vi "MainPannel.vi"() -> ()   [LabVIEW 2020]
uses:
  Digi/Digitizer_StatesMain.ctl
  <vilib>/userdefined/High Color/nirio_resource_hc.ctl
  Stage/New/StageOptions.ctl
  FileStore/Data Save State.ctl
  Gen/Generator_States.ctl
  <vilib>/Heliosphere Research LLC/Advanced Plotting Toolkit/properties/Colormap_Map.ctl
  <vilib>/Native 3D Graph/xcontrol/3DPC_SurfacePlot.xctl
  PixelImageState.ctl
  <vilib>/UPVI/lvhdf5/library.llb/HDF5 Ref.ctl
  WaveClusterPacket.ctl
  <vilib>/Platform/TimedLoop/XDataNode/timing_clust.ctl
  <vilib>/Platform/TimedLoop/XDataNode/nitl_modes.ctl
  <vilib>/Platform/TimedLoop/XDataNode/wakeup.ctl
  Stage/New/SettingCtrlOptions.ctl
  Stage/New/PosCtrlOptions.ctl
  Digi/Controls/FPGA VI Reference.ctl
  <extravilib>/ChannelInstances/Tag-bool/Read With Abort.vi
  <extravilib>/ChannelInstances/Tag-bool/Write.vi
  <extravilib>/ChannelInstances/Tag-bool/Write With Abort.vi
  <extravilib>/ChannelInstances/Tag-bool/Instantiate.vi
  <extravilib>/ChannelInstances/Tag-bool/EndpointRead.vi
  <vilib>/FPGAPlugInAG/PXIe-7962R/niLvFpga_Open_PXIe-7962R.vi
  <vilib>/rvi/interface/common/dynamic/niFpgaDynamicAddResources.vi
  <vilib>/FPGAPlugInAG/Dynamic/niLvFpga_Close_Dynamic.vi
  <extravilib>/ChannelInstances/Tag-bool/Endpoint.vi
  <instrlib>/_niInstr/Basic Elements/v1/FPGA/Private/Count Up U32.vi
  <vilib>/Platform/TimedLoop/XDataNode/XDataNode.xnode
  <vilib>/rvi/interface/nirviOpenFPGA/nirviOpenFPGA.xnode
  FPGA Bitfiles/DigitizerFPGACode(Fully_Functional)_v3.lvbitx
  <vilib>/rvi/interface/nirviCloseFPGA/nirviCloseFPGA.xnode
  <instrlib>/_niInstr/Basic Elements/v1/FPGA/niInstr Basic Elements v1 FPGA.lvlib
  <vilib>/Platform/TimedLoop/XDataNode/XDNodeRunTimeDep.lvlib
  Stage/libximc.lvlib
  <extravilib>/ChannelInstances/Tag-bool.lvlib
  <vilib>/Heliosphere Research LLC/Advanced Plotting Toolkit/Advanced Plotting Toolkit.lvlib
panel:
  in  "LogMode":bool
  in  "Start Digitizer UI Bttn":bool
  out "Max Index (s)":dbl format="%#_3p"
  out "Max Val (V)":dbl format="%#_3p"
  in  "Delay_Scroll_Range":dbl=2.0 caption="Range"
  in  "FineDelayControl":dbl(slide)=1.0 step=0.1 scale=-2.0..2.0
  in  "Amplitude Range":cluster{"Slider 1":dbl, "Slider 1":dbl}(slide)={"Slider 1"=1.0, "Slider 1"=1.6299559471365639} scale=-2.5..2.5
  in  "Pause Triggger":bool caption="Pause"
  in  "Delay(us)":sgl min=0 step=0.1 format="%#_4g"
  in  "Time Division":u8(slide)=1 max=2 step=1 scale=0.0..2.0
  in  "Amplitude \nAveraging":u16(slide)=1 caption="Amplitude Averaging" scale=0.0..7.0 scale format="%#.2g"
  in  "Record Size":u16=1024
  in  "RIO Resource":T1="PXI1Slot2"
  out "Configured?":bool
  out "TIS Configured?":bool
  out "Range (Vpp)":dbl=1.3
  out "Digitizer On":bool
  out "Waveform [LIVE]":cluster{"Start Time":dbl, dbl, ext[]}(graph)
  in  "TriggerDigi":bool
  in  "Scanning":bool
  in  "Single Shot":bool
  in  "LIVE":bool
  out "Topography Plot":refnum<class "Base Datatype.lvclass">[](xcontrol)
  in  "Axis":bool
  in  "ColorBar":bool
  in  "Map":T2
  out "Scanned Image":picture
  in  "Transducer Freq (Hz)":u64
  in  "Temperature (C)":dbl
  in  "Remarks":string
  in  "Immersion Medium":string
  in  "EXIT APP":bool
  in  "Save to File":bool=TRUE caption="Checkbox"
  out "No Trig Miss":bool
  in  "FileName":string
  in  "File Store Directory":path
  out "File Open?":bool
  out "X Step Size (R)":sgl format="%#_2g"
  out "Y Step Size (R)":sgl format="%#_2g"
  out "Scan Time (Approx.)":string
  out "Total Pixels":i32
  out "Moving?":bool
  out "Stage Position":cluster{sgl[], sgl[]}(graph) caption="XY Graph - Dark"
  in  "X Position Abs":dbl caption="X Position"
  in  "Y Position Abs":dbl caption="Y Position"
  out "Line Count":i32=6 caption="Y Pixels"
  out "Pixel Count":i32=6 caption="X Pixels"
  in  "X Start":sgl
  in  "X End":sgl=10.0
  in  "Y Start":sgl
  in  "Y End":sgl=8.0
  in  "Y Step Size":sgl=0.5
  in  "X Step Size":sgl=0.5
  in  "Scan Mode":enum16{"Raster", "Serpentine"}(ring)
  in  "Speed Control (mm/s)":sgl(slide)=4.0 min=0.1 scale=0.1..5.0
  in  "AbsMove":bool
  in  "Outline":bool
  in  "Start Stage":bool
  in  "Stop Motion":bool
  in  "Zero":bool
  in  "Right":bool
  in  "Left":bool
  in  "Move to Start":bool
  in  "Down":bool
  in  "Up":bool
  out "X Position":dbl format="%#.3g"
  out "Y Position":dbl format="%#.3g"
  in  "Move Step":dbl=1.0
  in  "Stop Stage":bool
  out "Controller Open?":bool
  in  "Tab Control":enum32{"Developer Options"}(tab)
  out "Scan Running":bool=TRUE
  in  "Next Coordinate Index":i32
  in  "EdgePt/nPixelMap":bool=TRUE
  out "Coordinate Array":sgl[][](array[numeric])
  out "Step Sizes":sgl[](array[numeric])
  out "Peripheral Coordis":sgl[][](array[numeric])=[[0.0, 0.0], [1.8, 0.0], [3.6, 0.0], [5.3999996, 0.0], [7.2, 0.0], [9.0, 0.0], [9.0, 2.0], [7.2, 2.0], [5.3999996, 2.0], [3.6, 2.0], [1.8, 2.0], [0.0, 2.0], [0.0, 4.0], [1.8, 4.0], [3.6, 4.0], [5.3999996, 4.0], [7.2, 4.0], [9.0, 4.0], [9.0, 6.0], [7.2, 6.0], [5.3999996, 6.0], [3.6, 6.0], [1.8, 6.0], [0.0, 6.0], [0.0, 8.0], [1.8, 8.0], [3.6, 8.0], [5.3999996, 8.0], [7.2, 8.0], [9.0, 8.0], [9.0, 10.0], [7.2, 10.0], [5.3999996, 10.0], [3.6, 10.0], [1.8, 10.0], [0.0, 10.0]]
  in  "Correction Table Path (Hidden)":path
  out "Serial nos":u32[](array[numeric])
  out "Calibration":cluster{dbl, "MicrostepMode":u32}[](array[cluster])
  out "IDs":i32[](array[numeric])
  in  "X Max Stage":dbl=220.0 format="%#_13g"
  in  "Y Maximum":dbl=220.0
  out "Stage Status":T3
  out "Waves Received":u32
  in  "reset Rx wave count":bool
  out "Digi State":T4
  out "nDigiLoopRunning":bool
  in  "Send vi Trig":bool
  out "Gain":dbl
  out "Offset Factor":dbl
  out "Amplitudes":dbl[](array[numeric]) format="%.2f"
  out "Sampling Frequency (Hz)":u64
  out "Waves per Pixel":u32
  in  "Ext/nViTrig":bool=TRUE
  out "FileStore State":T5
  out "Gen State":T6
  out "PixelMap_Scan":i32[][](array[numeric])
  out "error out Digi":errorcluster
  in  "Scan Started":bool
  out "Scan Complete":bool=TRUE
  out "Image State":T7
  out "Wave Count Zero":bool
  out "Error Out Gen":errorcluster
  in  "CountReset":bool
  in  "Stop Gen App":bool
  in  "Machine Mode":T8(ring)=enum."Normal"
  in  "Stop Stage App":bool
  in  "Trigger Digi Single":bool
  in  "Start Digi":bool
  in  "Stop Digi App":bool caption="Stop Digi \nApplication"
  in  "Digi Machine Mode":T9(ring)=enum."Single Shot Mode"
  in  "Done Recording":bool
  in  "Record Data":bool
  in  "Open File":bool
  in  "Stop File App":bool
  in  "Reset Img Ma":bool
  in  "Generator  Port":refnum<k15>
  out "Actual Sample Rate":dbl format="%#_6p"
  in  "Use Default Wave Settings":bool caption="Checkbox"
  in  "Start Gen":bool
  in  "stop Gen":bool
  out "Generator On":bool
  out "Input Waveform":dbl[](graph)
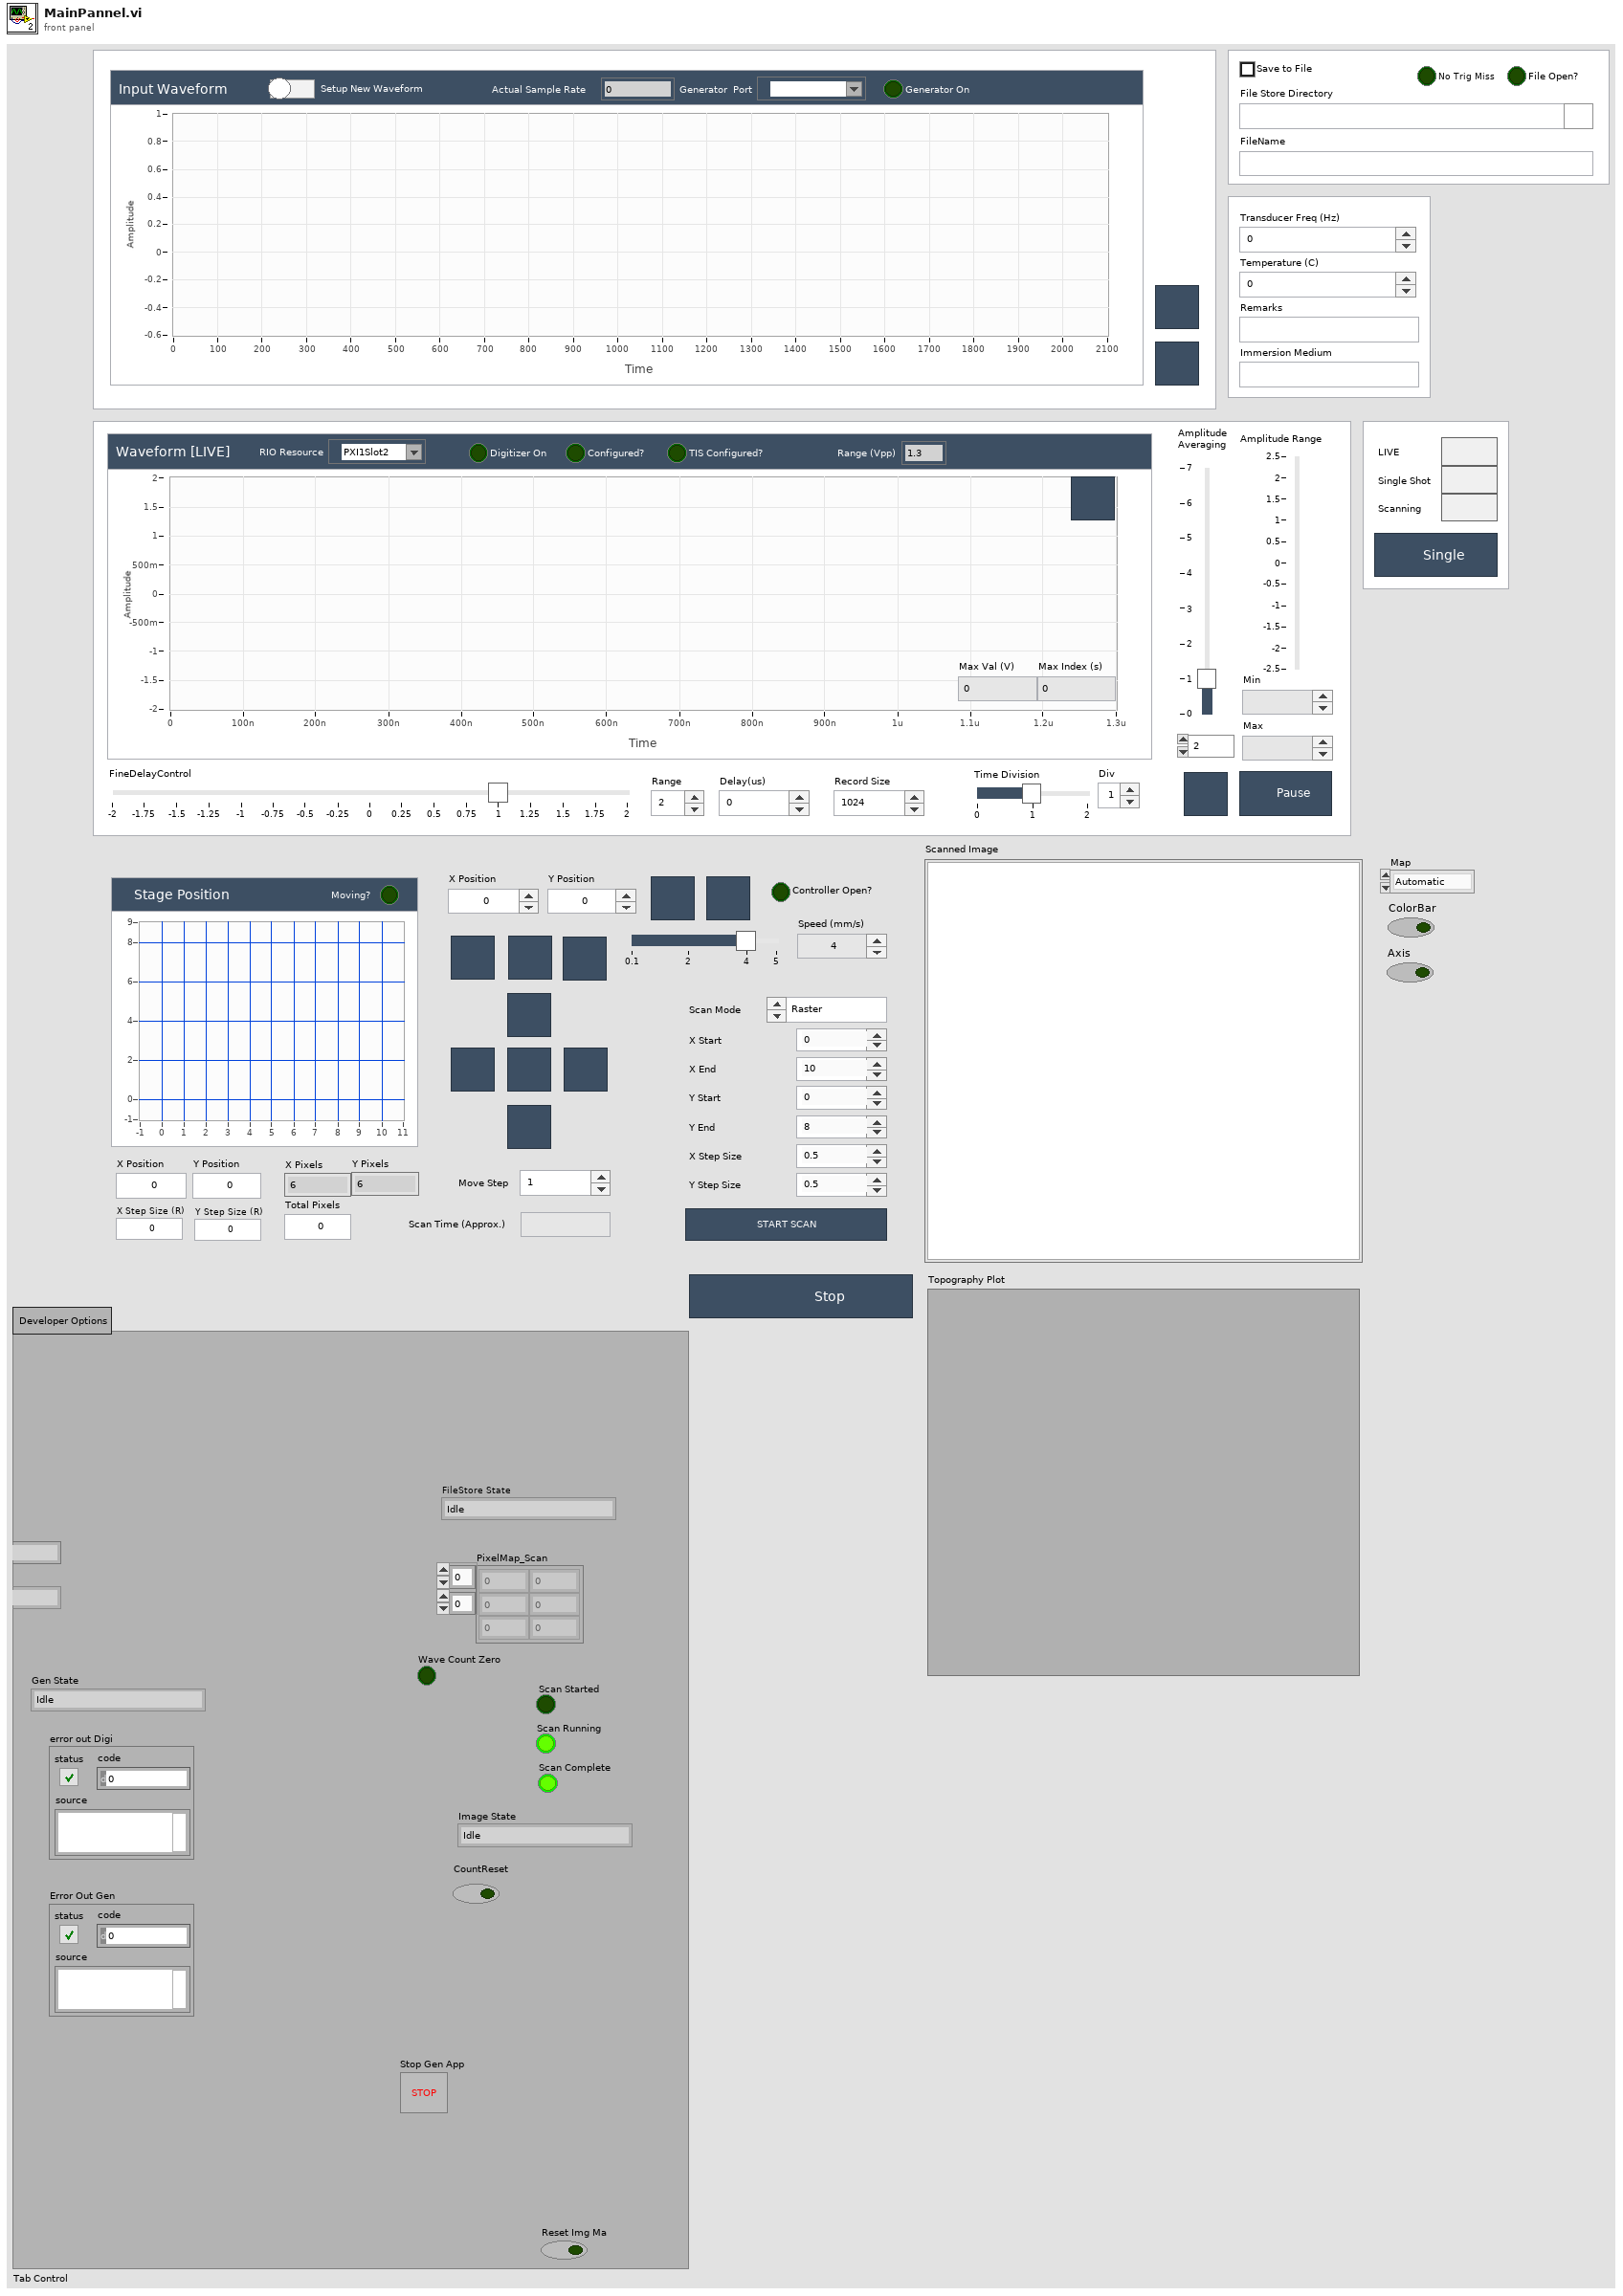
[diagram p1: front panel]
types:
  T1 = typedef "nirio_resource_hc.ctl" = tag
  T2 = typedef "Advanced Plotting Toolkit.lvlib/Colormap_Map.ctl" = enum16{"Automatic", "Rainbow", "Hot and Cold", "White-Black", "White-Blue", "White-Green", "White-Red", "Fire", "Water", "Earth", "Air", "Pastel", "Banded", "Stepped"}
  T3 = typedef "StageOptions.ctl" = enum16{"Idle", "Init", "Set Speed", "GenerateMotionPoints", "Scan_Start", "Scan_MoveNext", "Scan_SyncSet", "Scan_Get Pos", "Scan_Complete", "Cmd_MoveAbs", "Cmd_CloseControllers", "Cmd_MoveUp", "Cmd_MoveDown", "Cmd_MoveLeft", "Cmd_MoveRight", "Cmd_MoveStart", "Cmd_MoveZero", "Cmd_GetPos", "Cmd_Stop", "Sync_On", "Sync_Off", "Stop Motion", "CloseApplication"}
  T4 = typedef "Digitizer_StatesMain.ctl" = enum16{"Idle", "Init", "SetParam", "VITrig", "Read", "CloseDigi", "CloseApp"}
  T5 = typedef "Data Save State.ctl" = enum16{"Idle", "Open File", "Write Attributes", "Append Data", "Close File", "Close App"}
  T6 = typedef "Generator_States.ctl" = enum16{"Idle", "GenerateWaveArray", "InitGen", "SendVITrig", "CloseGen", "CloseApp"}
  T7 = typedef "PixelImageState.ctl" = enum16{"Idle", "Init", "Update Pixel", "Complete Imaging"}
  T8 = enum16{"Scanning Mode", "Perimeter Mode", "Normal"}
  T9 = enum16{"Scanning Mode", "Live Mode", "Single Shot Mode"}
  T10 = typedef "WaveClusterPacket.ctl" = cluster{"Wave Count":u32, "Wave":i16[]}
  T11 = typedef "HDF5 Ref.ctl" = refnum<k1>
  T12 = typedef "XDNodeRunTimeDep.lvlib/timing_clust.ctl" = cluster{"Expected End [f-1]":u64, "Actual End [f-1]":u64, "Finished Late? [f-1]":bool, "Expected End [i-1]":u64, "Actual End [i-1]":u64, "Finished Late? [i-1]":bool, "Expected Start [i]":u64, "Actual Start [i]":u64, "Expected Start [f]":u64, "Actual Start [f]":u64, "Source Name":string, "Structure Name":string, "Period":i64, "Deadline":i64, "Offset":i64, "Start":i64, "Priority":i32, "Timeout":i32, "Mode":T13, "Wakeup Reason":T14, "Error":errorcluster, "Source Type":string, "Secondary Source Type":string, "Global End Time":u64, "Global Start Time":u64, "Frame Duration":u64, "Iteration Duration":u64, "Assigned CPU":i32, "I/O Scan Engine Mode":u32}
  T13 = typedef "XDNodeRunTimeDep.lvlib/nitl_modes.ctl" = enum32{"No Change", "Process missed periods, maintain original phase", "Discard missed periods, maintain original phase", "Process missed periods, ignore original phase", "Discard missed periods, ignore original phase"}
  T14 = typedef "XDNodeRunTimeDep.lvlib/wakeup.ctl" = enum32{"Normal", "Aborted", "Asynchronous wakeup", "Timing source error", "Timed loop error", "Timeout"}
  T15 = typedef "SettingCtrlOptions.ctl" = enum16{"Set X", "Set Y", "Set X and Y", "Get Settings", "None"}
  T16 = typedef "PosCtrlOptions.ctl" = enum16{"Move X", "Move Y", "Both X and Y", "Read Pos", "None"}
  T17 = typedef "FPGA VI Reference.ctl" = refnum<k20>
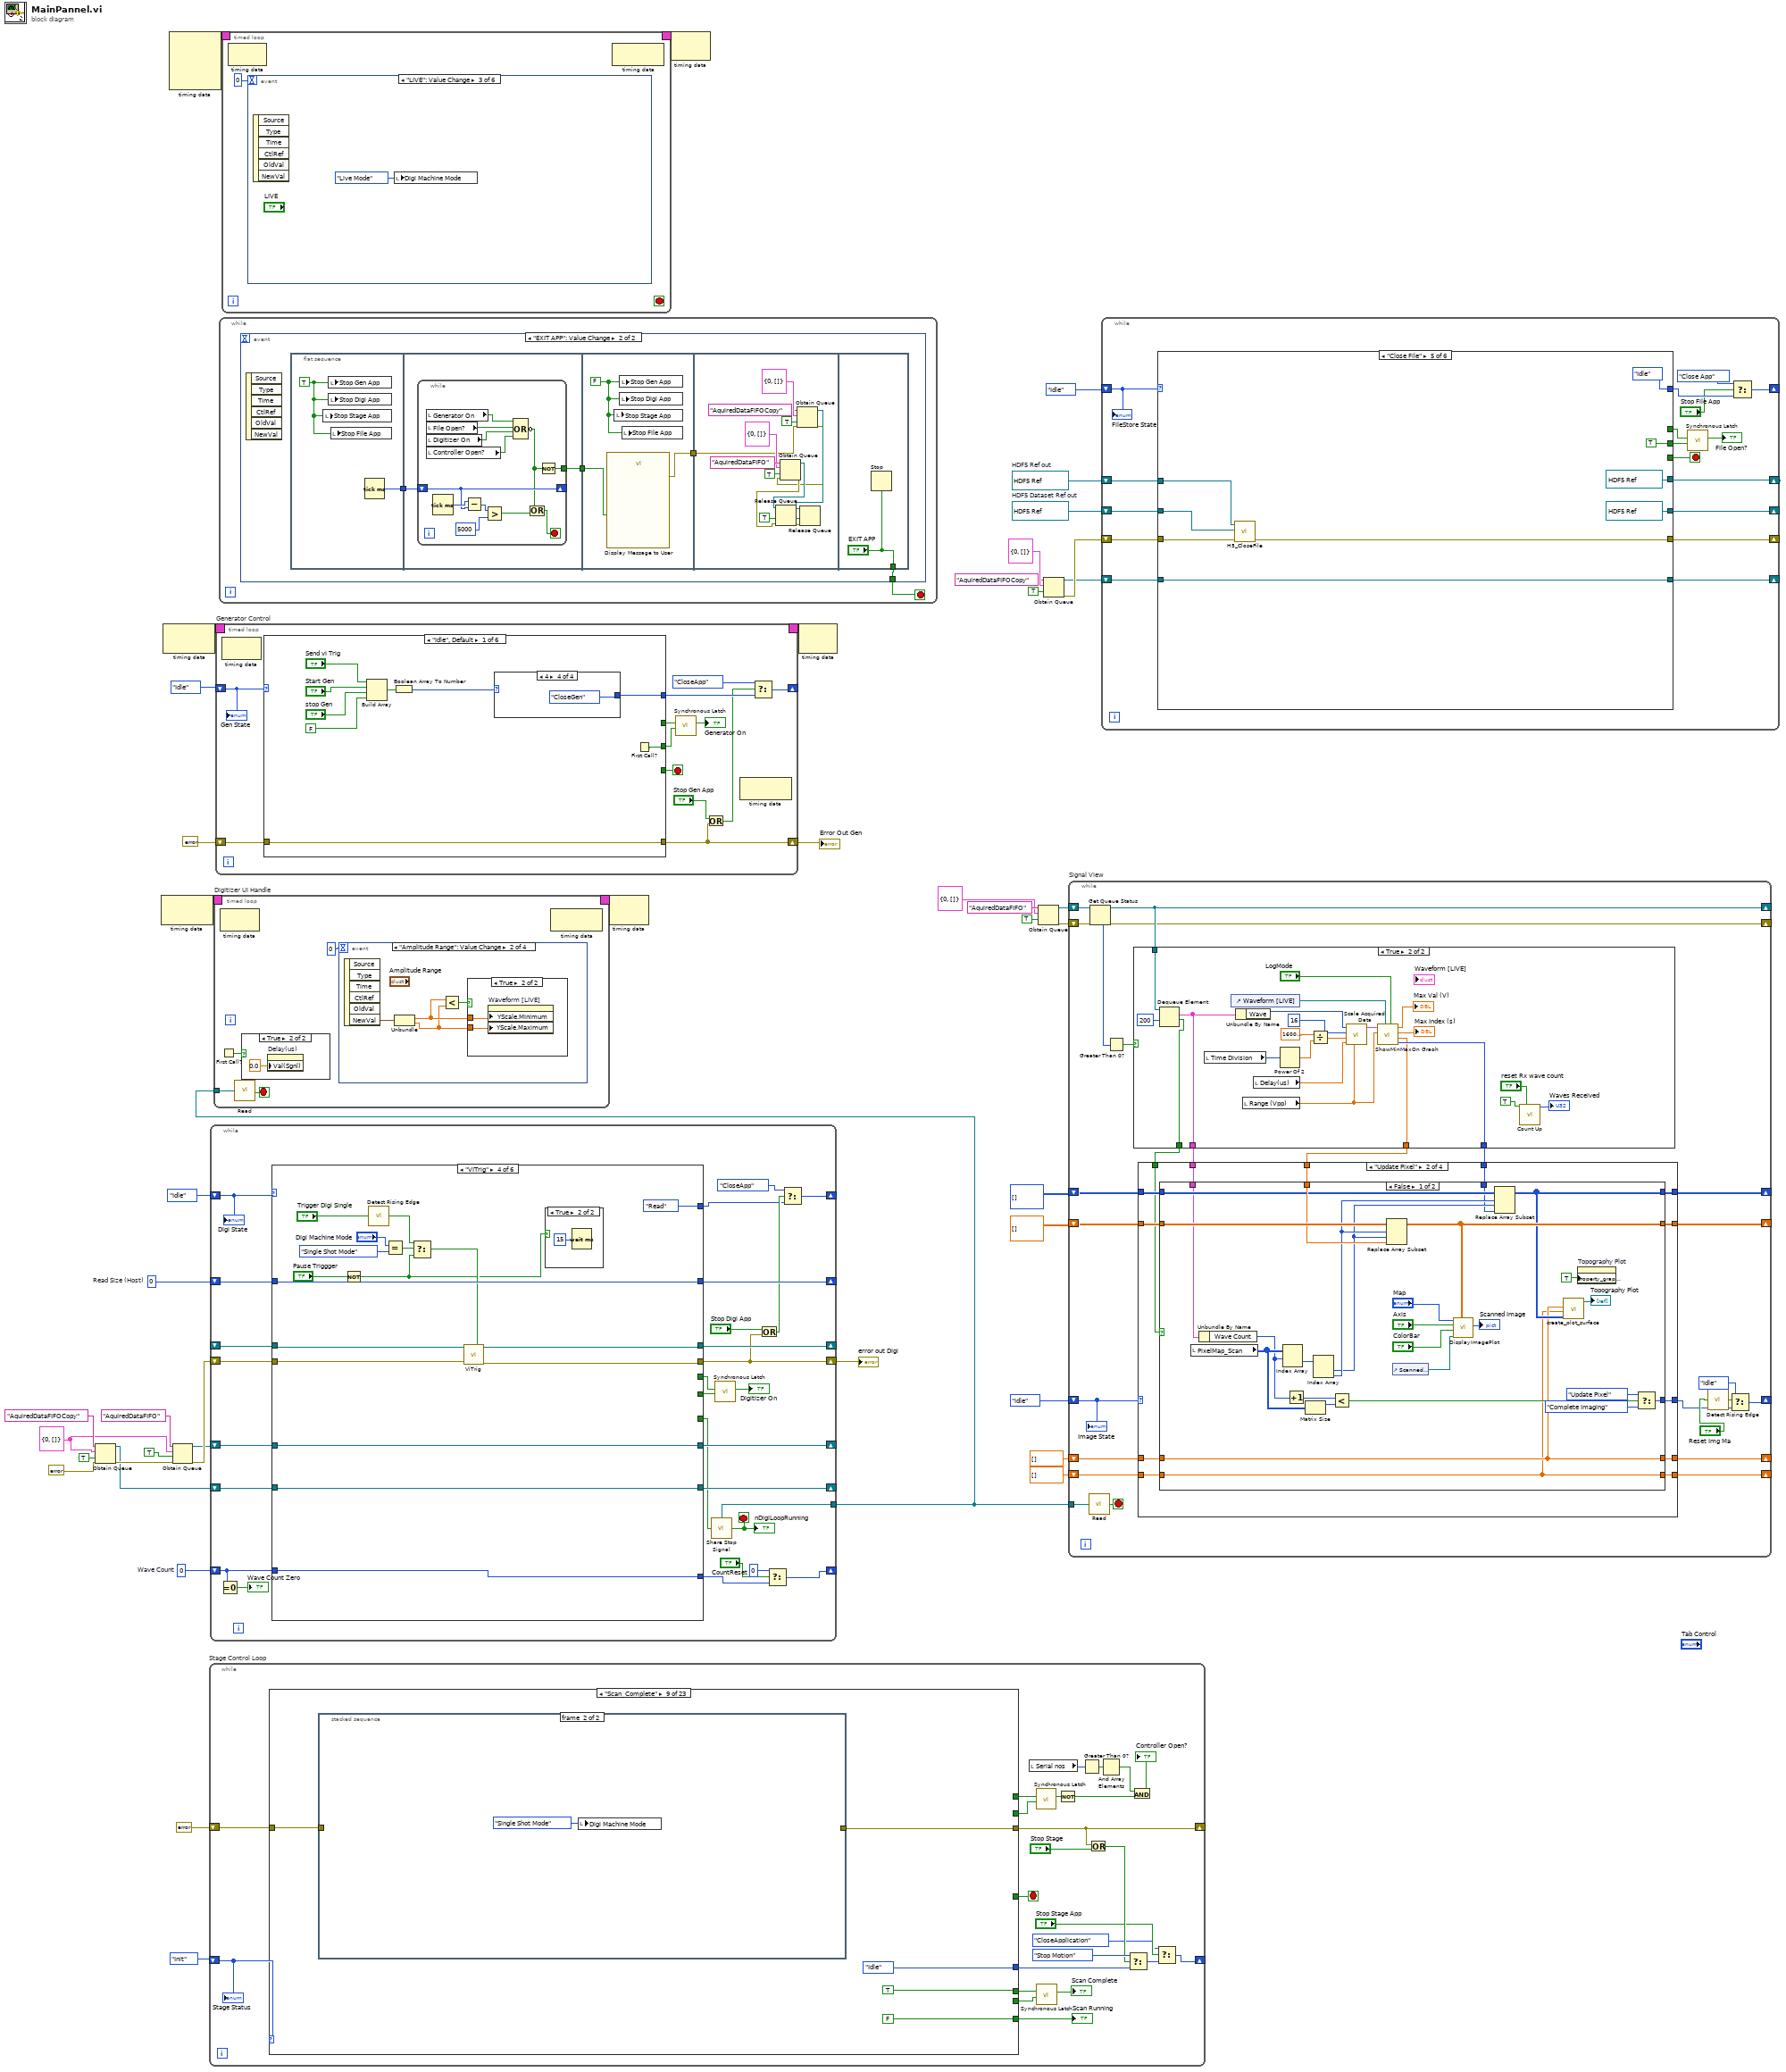
[diagram p0: block diagram]
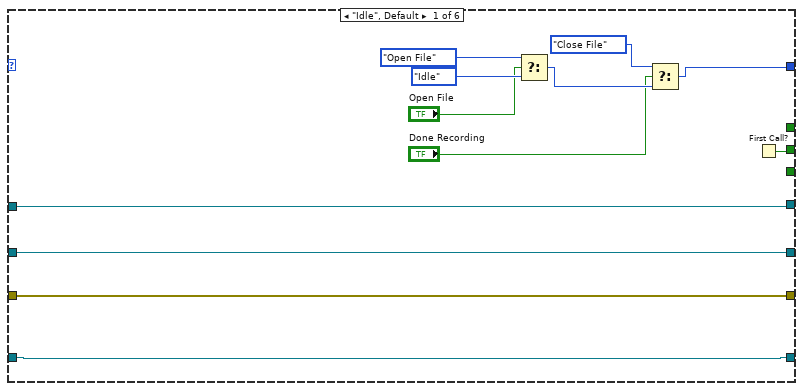
[diagram p2: hidden frame]
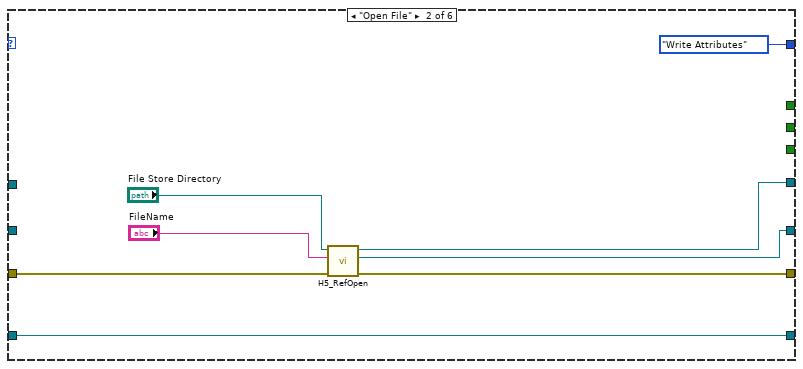
[diagram p3: hidden frame]
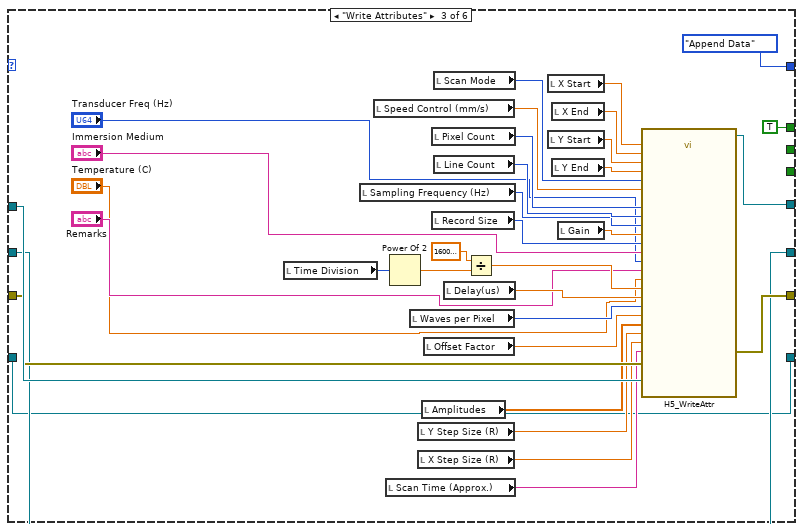
[diagram p4: hidden frame]
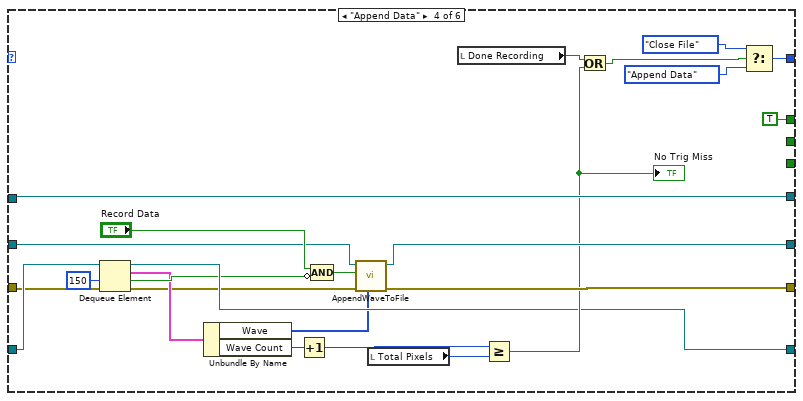
[diagram p5: hidden frame]
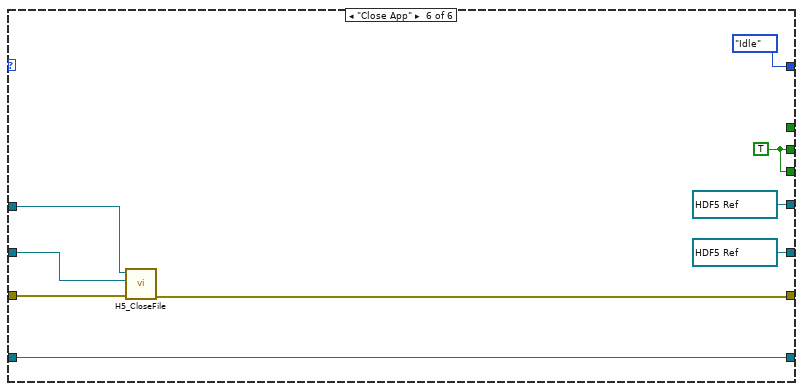
[diagram p6: hidden frame]
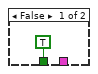
[diagram p7: hidden frame]
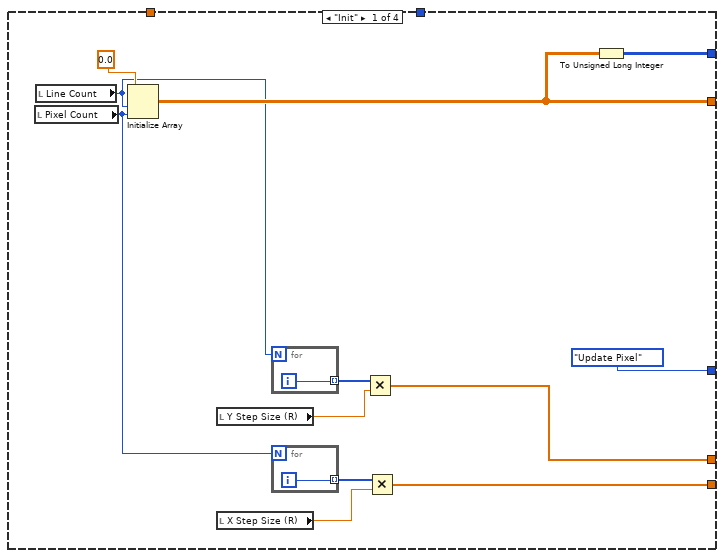
[diagram p8: hidden frame]
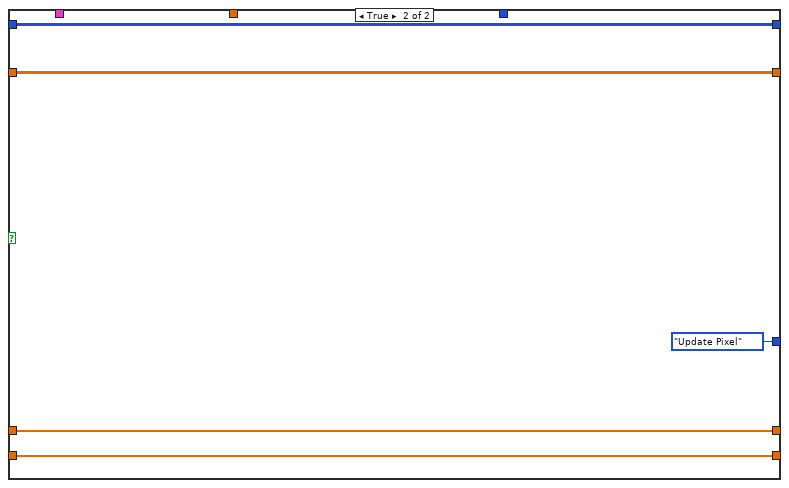
[diagram p9: hidden frame]
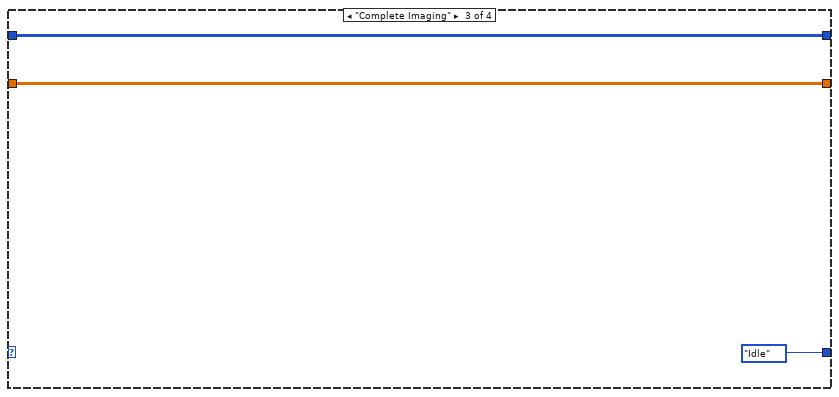
[diagram p10: hidden frame]
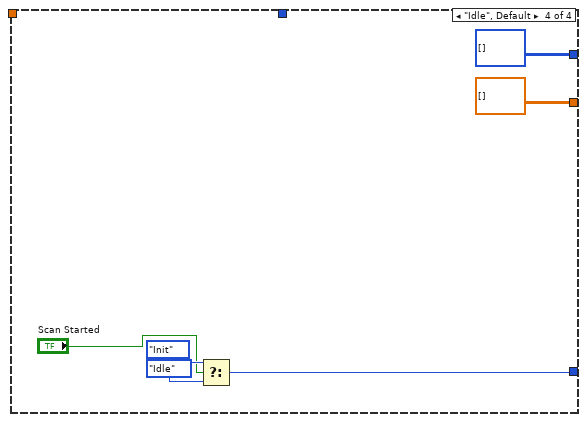
[diagram p11: hidden frame]
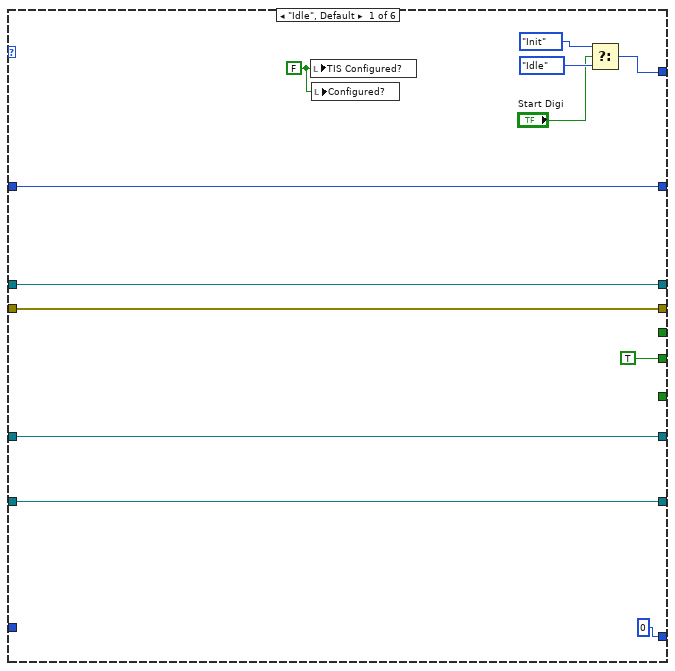
[diagram p12: hidden frame]
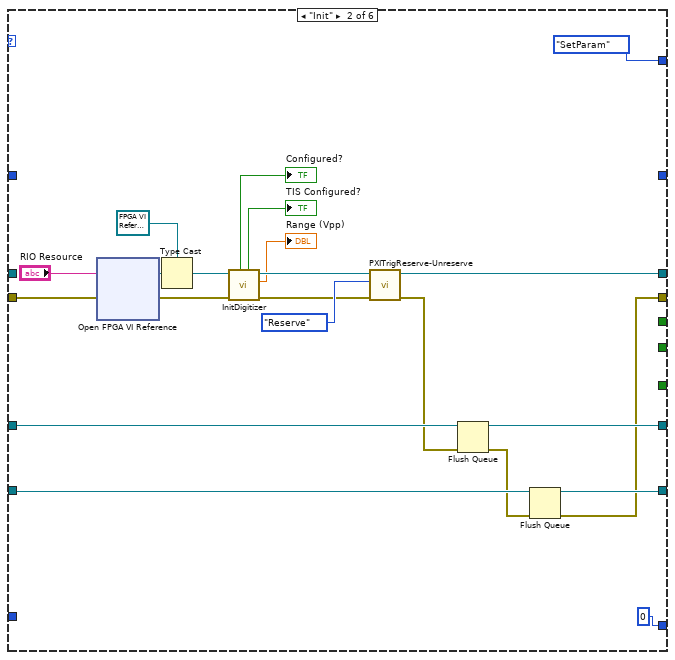
[diagram p13: hidden frame]
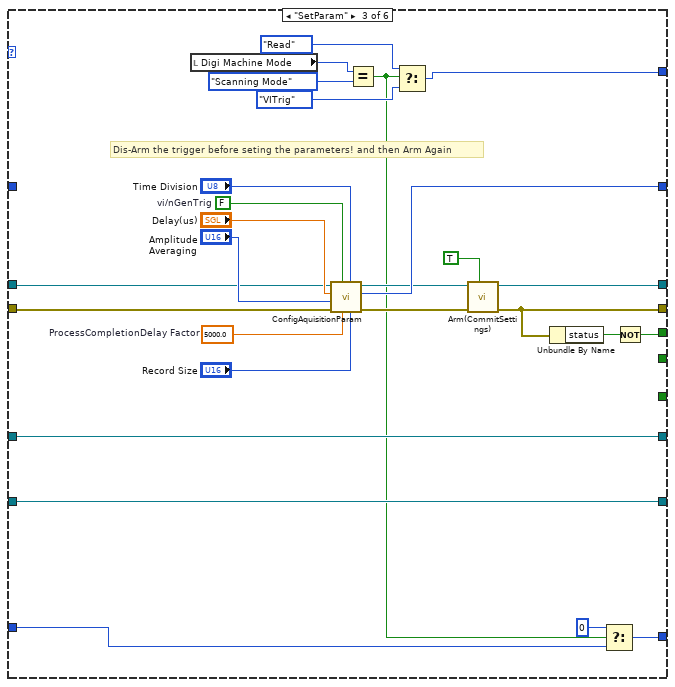
[diagram p14: hidden frame]
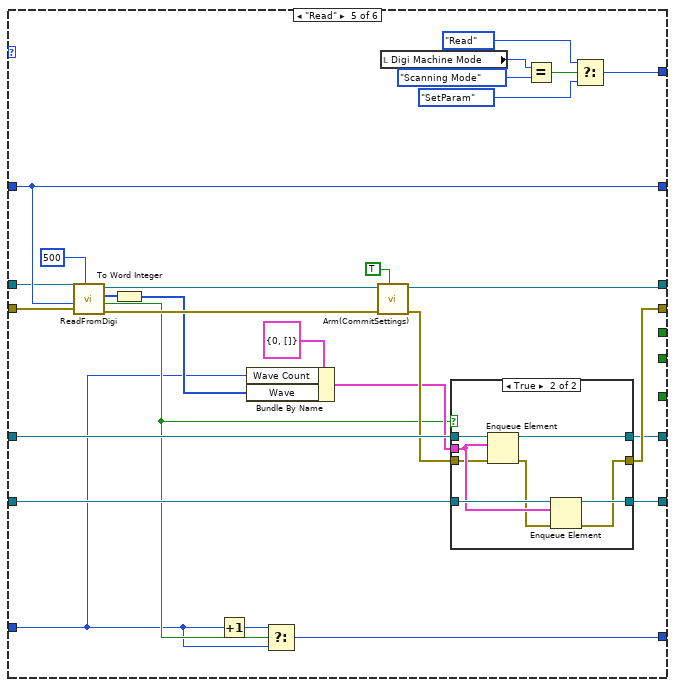
[diagram p16: hidden frame]
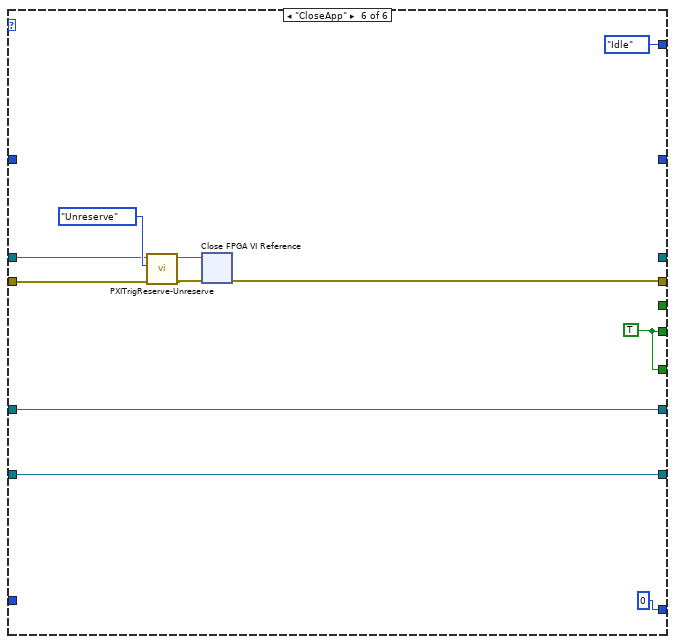
[diagram p18: hidden frame]
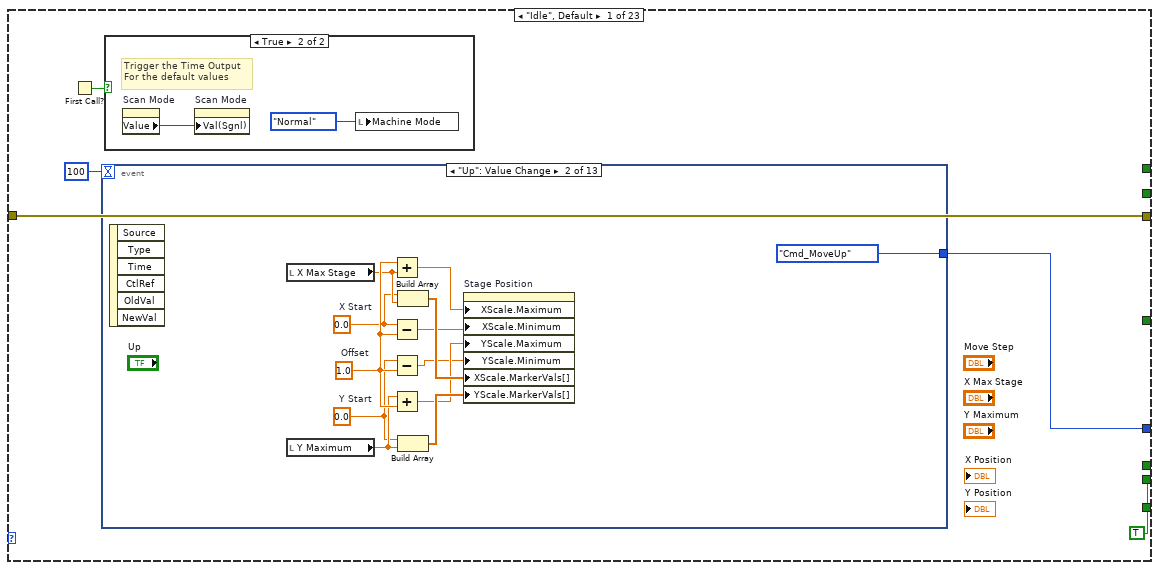
[diagram p19: hidden frame]
diagram:
  w12 = u16 0  # Wave Count
  w14 = T10 {"Wave Count"=0, "Wave"=[]} ("input cluster")
  w21 = T11 refnum items=["HDF5 Ref"]  # HDF5 Dataset Ref out
  w22 = T11 refnum items=["HDF5 Ref"]  # HDF5 Ref out
  w39 = u16 0  # Read Size (Host)
  n1 = Obtain Queue(name (unnamed)="AquiredDataFIFOCopy", element data type=w14, create if not found? (T)=TRUE, error in (no error)=errorcluster {"status"=FALSE, "code"=0, "source"=""}) -> (queue out=w16:refnum<queue>, error out=w17:errorcluster)  [unwired: 1 in, 1 out]
  n2 = node-c288() -> (w42:T12)  [unwired: 1 in]
  n3 = node-c288() -> (w36:T12)  [unwired: 1 in]
  n4 = node-c288() -> (w5:T12)  [unwired: 4 in]
  n5 = Obtain Queue(name (unnamed)="AquiredDataFIFO", element data type=w14, create if not found? (T)=TRUE, error in (no error)=w17) -> (queue out=w28:refnum<queue>, error out=w29:errorcluster)  [unwired: 1 in, 1 out]
  n6 = while "Stage Control Loop" {
    shift-right: [w57] -> _
    shift-left: StageOptions."Init" -> [w68]
    shift-right: [w65] -> _
    shift-left: errorcluster {"status"=FALSE, "code"=0, "source"=""} ("error out") -> [w66]
    stop <- w58 stop-if-true
    n7 = case shown="\"Scan_Complete\"" w68 {
      tunnel: [w73 w169 w192 w228 w233 w362 w377 w391 w431 w454 w463 w470 w481 w491 w501 w510 w518 w533 w539 w550 w559 w567 w578] -> w65
      tunnel: w66 -> [w73 w167 w193 w227 w235 w363 w378 w392 w429 w455 w464 w469 w482 w492 w502 w511 w519 w534 w538 w551 w560 w566 w577]
      tunnel: [w72 StageOptions."Set Speed" StageOptions."GenerateMotionPoints" w212 w236 w353 StageOptions."Scan_MoveNext" w388 StageOptions."Idle" StageOptions."Idle" StageOptions."Idle" StageOptions."Idle" StageOptions."Idle" StageOptions."Idle" StageOptions."Idle" StageOptions."Idle" StageOptions."Idle" StageOptions."Idle" StageOptions."Idle" StageOptions."Idle" StageOptions."Idle" StageOptions."Idle" StageOptions."Idle"] -> w63
      tunnel: [_ _ _ _ _ _ _ _ _ _ _ _ _ _ _ _ _ _ _ _ _ w563 w573] -> w61
      tunnel: [_ w170 _ _ _ _ _ _ _ _ _ _ _ _ _ _ _ _ _ _ _ _ _] -> w59
      tunnel: [_ _ _ _ _ _ _ _ _ _ _ _ _ _ _ _ _ _ _ _ _ _ w573] -> w58
      tunnel: [_ _ _ _ _ _ _ _ TRUE ("X SyncOut Enabled") _ _ _ _ _ _ _ _ _ _ _ _ _ _] -> w48
      tunnel: [TRUE ("EdgePt/nPixelMap") TRUE ("EdgePt/nPixelMap") TRUE ("EdgePt/nPixelMap") TRUE ("EdgePt/nPixelMap") TRUE ("EdgePt/nPixelMap") _ _ _ _ _ _ _ _ _ _ _ _ _ _ _ _ _ _] -> w46
      tunnel: [_ _ _ _ _ TRUE ("Moving?") TRUE ("Moving?") w379 FALSE ("Moving?") _ _ _ _ _ _ _ _ _ _ _ _ _ _] -> w45
      frame "Idle", Default {
        n8 = First Call?() -> (First Call?: T/F=w70:bool)
        n9 = event shown="[1] \"Up\": Value Change" {
          selector: _ -> [_ _ _ _ _ _ _ _ _ _ _ _ _]
          dyn-events: _ -> [_ _ _ _ _ _ _ _ _ _ _ _ _]
          timeout: 100 -> [_ _ _ _ _ _ _ _ _ _ _ _ _]
          tunnel: [w76 StageOptions."Cmd_MoveUp" StageOptions."Cmd_MoveDown" StageOptions."Cmd_MoveStart" StageOptions."Cmd_MoveLeft" StageOptions."Cmd_MoveRight" StageOptions."Cmd_MoveZero" StageOptions."Cmd_Stop" StageOptions."GenerateMotionPoints" StageOptions."GenerateMotionPoints" StageOptions."Set Speed" w148 StageOptions."Cmd_MoveAbs"] -> w72
          event Timeout {
            n10 = event-data() -> ()  [unwired: 1 in, 3 out]
            n11 = local read "Controller Open?"() -> (w77:bool)
            n12 = case shown="False" w77 {
              tunnel: [StageOptions."Init" StageOptions."Cmd_GetPos"] -> w76
              frame False {
              }
              frame True {
              }
            }
          }
          event "Up": Value Change {
            w80 = 0.0  # Y Start
            w82 = sgl 0.0  # X Start
            w85 = 1.0  # Offset
            n13 = event-data() -> ()  [unwired: 1 in, 6 out]
            n14 = local read "X Max Stage"() -> (w83:dbl)
            n15 = local read "Y Maximum"() -> (w81:dbl)
            n16 = Add(x=w85, y=w83) -> (x+y=w87:dbl)
            n17 = Subtract(x=w82, y=w85) -> (x-y=w88:dbl)
            n18 = Subtract(x=w80, y=w85) -> (x-y=w84:dbl)
            n19 = Add(x=w81, y=w85) -> (x+y=w86:dbl)
            n20 = Build Array(w82, w83) -> (w90:dbl[])
            n21 = Build Array(w80, w81) -> (w89:dbl[])
            n22 = property on="Stage Position" class="XYGraph (strict)"("XScale.Maximum"=w87, "XScale.Minimum"=w88, "YScale.Maximum"=w86, "YScale.Minimum"=w84, "XScale.MarkerVals[]"=w90, "YScale.MarkerVals[]"=w89) -> ()  [unwired: 2 in, 2 out]
          }
          event "Down": Value Change {
            w92 = 0.0  # Y Start
            w94 = sgl 0.0  # X Start
            w97 = 1.0  # Offset
            n23 = event-data() -> ()  [unwired: 1 in, 6 out]
            n24 = local read "X Max Stage"() -> (w95:dbl)
            n25 = local read "Y Maximum"() -> (w93:dbl)
            n26 = Add(x=w97, y=w95) -> (x+y=w99:dbl)
            n27 = Subtract(x=w94, y=w97) -> (x-y=w100:dbl)
            n28 = Subtract(x=w92, y=w97) -> (x-y=w96:dbl)
            n29 = Add(x=w93, y=w97) -> (x+y=w98:dbl)
            n30 = Build Array(w94, w95) -> (w102:dbl[])
            n31 = Build Array(w92, w93) -> (w101:dbl[])
            n32 = property on="Stage Position" class="XYGraph (strict)"("XScale.Maximum"=w99, "XScale.Minimum"=w100, "YScale.Maximum"=w98, "YScale.Minimum"=w96, "XScale.MarkerVals[]"=w102, "YScale.MarkerVals[]"=w101) -> ()  [unwired: 2 in, 2 out]
          }
          event "Move to Start": Value Change {
            n33 = event-data() -> ()  [unwired: 1 in, 6 out]
          }
          event "Left": Value Change {
            w105 = 0.0  # Y Start
            w107 = sgl 0.0  # X Start
            w110 = 1.0  # Offset
            n34 = event-data() -> ()  [unwired: 1 in, 6 out]
            n35 = local read "X Max Stage"() -> (w108:dbl)
            n36 = local read "Y Maximum"() -> (w106:dbl)
            n37 = Add(x=w110, y=w108) -> (x+y=w112:dbl)
            n38 = Subtract(x=w107, y=w110) -> (x-y=w113:dbl)
            n39 = Subtract(x=w105, y=w110) -> (x-y=w109:dbl)
            n40 = Add(x=w106, y=w110) -> (x+y=w111:dbl)
            n41 = Build Array(w107, w108) -> (w115:dbl[])
            n42 = Build Array(w105, w106) -> (w114:dbl[])
            n43 = property on="Stage Position" class="XYGraph (strict)"("XScale.Maximum"=w112, "XScale.Minimum"=w113, "YScale.Maximum"=w111, "YScale.Minimum"=w109, "XScale.MarkerVals[]"=w115, "YScale.MarkerVals[]"=w114) -> ()  [unwired: 2 in, 2 out]
          }
          event "Right": Value Change {
            w117 = 0.0  # Y Start
            w119 = sgl 0.0  # X Start
            w122 = 1.0  # Offset
            n44 = event-data() -> ()  [unwired: 1 in, 6 out]
            n45 = local read "X Max Stage"() -> (w120:dbl)
            n46 = local read "Y Maximum"() -> (w118:dbl)
            n47 = Add(x=w122, y=w120) -> (x+y=w124:dbl)
            n48 = Subtract(x=w119, y=w122) -> (x-y=w125:dbl)
            n49 = Subtract(x=w117, y=w122) -> (x-y=w121:dbl)
            n50 = Add(x=w118, y=w122) -> (x+y=w123:dbl)
            n51 = Build Array(w119, w120) -> (w127:dbl[])
            n52 = Build Array(w117, w118) -> (w126:dbl[])
            n53 = property on="Stage Position" class="XYGraph (strict)"("XScale.Maximum"=w124, "XScale.Minimum"=w125, "YScale.Maximum"=w123, "YScale.Minimum"=w121, "XScale.MarkerVals[]"=w127, "YScale.MarkerVals[]"=w126) -> ()  [unwired: 2 in, 2 out]
          }
          event "Zero": Value Change {
            w129 = 0.0  # Y Start
            w131 = sgl 0.0  # X Start
            w134 = 1.0  # Offset
            n54 = event-data() -> ()  [unwired: 1 in, 6 out]
            n55 = local read "X Max Stage"() -> (w132:dbl)
            n56 = local read "Y Maximum"() -> (w130:dbl)
            n57 = Add(x=w134, y=w132) -> (x+y=w136:dbl)
            n58 = Subtract(x=w131, y=w134) -> (x-y=w137:dbl)
            n59 = Subtract(x=w129, y=w134) -> (x-y=w133:dbl)
            n60 = Add(x=w130, y=w134) -> (x+y=w135:dbl)
            n61 = Build Array(w131, w132) -> (w139:dbl[])
            n62 = Build Array(w129, w130) -> (w138:dbl[])
            n63 = property on="Stage Position" class="XYGraph (strict)"("XScale.Maximum"=w136, "XScale.Minimum"=w137, "YScale.Maximum"=w135, "YScale.Minimum"=w133, "XScale.MarkerVals[]"=w139, "YScale.MarkerVals[]"=w138) -> ()  [unwired: 2 in, 2 out]
          }
          event "Stop Motion": Value Change {
            n64 = event-data() -> ()  [unwired: 1 in, 6 out]
          }
          event "Start Stage": Value Change {
            n65 = event-data() -> ()  [unwired: 1 in, 6 out]
            n66 = local write "Machine Mode"(T8."Scanning Mode" ("Machine Mode")) -> ()
          }
          event "X Start", "X End", "Y Start", "Y End", "Y Step Size", "X Step Size", "Scan Mode": Value Change {
            n67 = event-data() -> ()  [unwired: 1 in, 6 out]
            n68 = local write "Machine Mode"(T8."Normal" ("Machine Mode")) -> ()
          }
          event "Speed Control (mm/s)": Value Change {
            n69 = event-data() -> ()  [unwired: 1 in, 6 out]
          }
          event "Outline": Value Change {
            n70 = event-data() -> ()  [unwired: 1 in, 6 out]
            n71 = case shown="True" "Outline" {
              tunnel: [StageOptions."Idle" StageOptions."GenerateMotionPoints"] -> w148
              frame False {
              }
              frame True {
                n72 = local write "Machine Mode"(T8."Perimeter Mode" ("Machine Mode")) -> ()
              }
            }
          }
          event "AbsMove": Value Change {
            w152 = 0.0  # Y Start
            w154 = sgl 0.0  # X Start
            w157 = 1.0  # Offset
            n73 = event-data() -> ()  [unwired: 1 in, 6 out]
            n74 = local read "X Max Stage"() -> (w155:dbl)
            n75 = local read "Y Maximum"() -> (w153:dbl)
            n76 = Add(x=w157, y=w155) -> (x+y=w159:dbl)
            n77 = Subtract(x=w154, y=w157) -> (x-y=w160:dbl)
            n78 = Subtract(x=w152, y=w157) -> (x-y=w156:dbl)
            n79 = Add(x=w153, y=w157) -> (x+y=w158:dbl)
            n80 = Build Array(w154, w155) -> (w162:dbl[])
            n81 = Build Array(w152, w153) -> (w161:dbl[])
            n82 = property on="Stage Position" class="XYGraph (strict)"("XScale.Maximum"=w159, "XScale.Minimum"=w160, "YScale.Maximum"=w158, "YScale.Minimum"=w156, "XScale.MarkerVals[]"=w162, "YScale.MarkerVals[]"=w161) -> ()  [unwired: 2 in, 2 out]
          }
        }
        n83 = case shown="True" w70 {
          frame False {
          }
          frame True {
            # "Trigger the Time Output\nFor the default values"
            n84 = property on="Scan Mode" class="Enum (strict)"() -> ("Value"=w75:enum16{"Raster", "Serpentine"})  [unwired: 2 in, 2 out]
            n85 = property on="Scan Mode" class="Enum (strict)"("Val(Sgnl)"=w75) -> ()  [unwired: 2 in, 2 out]
            n86 = local write "Machine Mode"(T8."Normal" ("Machine Mode")) -> ()
          }
        }
      }
      frame "Init" {
        w176 = 100  # numSteps = 1mm
        w177 = TRUE  # Correction File Path Option
        n87 = call "CloseDevices.vi"("error in (no error)"=w167, "Close"=TRUE, "Ids"=i32[] [1, 2]) -> ("error out"=w166:errorcluster)  [unwired: 8 in]
        n88 = case shown="False" w177 {
          tunnel: ["Correction Table Path (Hidden)" w183] -> w178
          frame False {
          }
          frame True {
            w184 = path "Corr_table_8MT173-25.tbl"  # File Name
            n89 = Current VI's Path() -> (path=w186:path)
            n90 = Build Path(base path=w186, name or relative path=path "") -> (appended path=w185:path)
            n91 = Build Path(base path=w185, name or relative path=w184) -> (appended path=w183:path)
          }
        }
        n92 = call "Find Controllers.vi"("error in (no error)"=w166) -> ("error out"=w180:errorcluster, "Names"=w181:string[])  [unwired: 8 in, 1 out]
        n93 = call "OpenDevices.vi"("error In"=w180, "Names"=w181) -> ("error out"=w179:errorcluster, "Serial nos"=→"Serial nos":u32[], "IDs"=w174:i32[])  [unwired: 6 in]
        "IDs" <- w174
        n94 = call "CalibrateStage.vi"("error in (no error)"=w179, "numSteps = 1mm"=w176, "Correction Table Path"=w178, "IDs"=w174) -> ("error out"=w169:errorcluster, "Calibration"=→"Calibration":cluster{dbl, "MicrostepMode":u32}[])  [unwired: 2 in, 4 out]
        n95 = Unbundle By Name(w169) -> ("status"=w171:bool)
        n96 = Not(x=w171) -> (.not. x?=w170:bool)
      }
      frame "Set Speed" {
        n97 = local read "IDs"() -> (w191:i32[])
        n98 = local read "Calibration"() -> (w190:cluster{dbl, "MicrostepMode":u32}[])
        n99 = call "SetMoveSettings.vi"("Mode"=SettingCtrlOptions."Set X and Y", "error in (no error)"=w193, "Calibration"=w190, "Speed"="Speed Control (mm/s)", "IDs"=w191) -> ("error out"=w192:errorcluster)  [unwired: 4 in, 2 out]
      }
      frame "GenerateMotionPoints" {
        n100 = local read "Calibration"() -> (w218:cluster{dbl, "MicrostepMode":u32}[])
        n101 = Subtract(x="X End", y="X Start") -> (x-y=w207:sgl)
        n102 = Divide(x=w207, y="X Step Size") -> (x/y=w223:sgl)
        n103 = Subtract(x="Y End", y="Y Start") -> (x-y=w205:sgl)
        n104 = Increment(x=w223) -> (x+1=w210:sgl)
        n105 = Divide(x=w205, y="Y Step Size") -> (x/y=w220:sgl)
        n106 = To Long Integer(number=w210) -> (32bit integer=w222:i32)
        n107 = Increment(x=w220) -> (x+1=w209:sgl)
        n108 = To Long Integer(number=w209) -> (32bit integer=w219:i32)
        n109 = call "GenerateScanEndPts.vi"("X Start"="X Start", "Mode"="Scan Mode", "Calibration In"=w218, "X End"="X End", "Y Start"="Y Start", "Y End"="Y End", "error in"=w227, "Line Count"=w219, "Pixel Count"=w222, "EdgePt/nPixelMap"="EdgePt/nPixelMap") -> ("Coordinate Array"=→"Coordinate Array":sgl[][], "X Pixel Count"=w200:i32, "Step Sizes"=w202:sgl[], "Y Pixel Count"=w199:i32, "error out"=w228:errorcluster)  [unwired: 1 in]
        "Line Count" <- w199
        "Pixel Count" <- w200
        "Step Sizes" <- w202
        n110 = call "PeripheralCoordinates.vi"("Y End"="Y End", "Y Start"="Y Start", "X End"="X End", "X Start"="X Start") -> ("Coordinate Array"=→"Peripheral Coordis":sgl[][])  [unwired: 7 in]
        n111 = local read "Speed Control (mm/s)"() -> (w203:sgl)
        n112 = Multiply(x=w199, y=w200) -> (x*y=→"Total Pixels":i32)
        n113 = Index Array(array=w202) -> (element #1=→"X Step Size (R)":sgl, element #2=→"Y Step Size (R)":sgl)  [unwired: 2 in]
        n114 = call "Calculate Scan Time.vi"("Step Sizes"=w202, "Scan Mode"="Scan Mode", "Speed Control (mm/s)"=w203, "Line Count"=w199, "Pixel Count"=w200) -> ("TimeString"=→"Scan Time (Approx.)":string)  [unwired: 2 in, 4 out]
        n115 = call "GenerateScanPixelMap.vi"("Mode"="Scan Mode", "Line Count"=w199, "Pixel Count"=w200) -> ("Coordinate Array"=→"PixelMap_Scan":i32[][])  [unwired: 7 in, 1 out]
        n116 = case shown="\"Scanning Mode\"" "Machine Mode" {
          tunnel: [StageOptions."Scan_Start" StageOptions."Scan_Start" StageOptions."Idle"] -> w212
          frame "Scanning Mode" {
          }
          frame "Perimeter Mode" {
          }
          frame "Normal", Default {
          }
        }
      }
      frame "Scan_Start" {
        n117 = call <vilib>:"Set Busy.vi"("error in (no error)"=w235) -> ("error out"=w234:errorcluster)  [unwired: 9 in, 1 out]
        n118 = stacked-sequence {
          seq-local: [_ w244 _ _ _ _ _] -> [_ _ _ _ _ _ w315]
          seq-local: [w238 _ _ _ _ _ _] -> [_ _ _ _ _ _ w316]
          seq-local: [_ _ _ _ w297 _ _] -> [_ _ _ _ _ _ w313]
          seq-local: [_ _ _ w274 _ _ _] -> [_ _ _ _ _ _ w314]
          seq-local: [_ _ _ _ _ w306 _] -> [_ _ _ _ _ _ w311]
          tunnel: w234 -> [_ _ _ _ _ _ w335]
          tunnel: [_ _ _ _ _ _ w329] -> w237
          tunnel: [_ _ _ _ _ _ w318] -> w236
          frame #0 {
            # "Start Generator"
            n119 = control-ref of="stop Gen"() -> (w240:refnum<vi>)
            n120 = control-ref of="Generator On"() -> (w242:refnum<vi>)
            n121 = control-ref of="Start Gen"() -> (w241:refnum<vi>)
            n122 = call "SwitchTillOn.vi"("Stop if On?"=TRUE, "Turn Off Button"=w240, "timeout"=u32 5000, "Turn On Button"=w241, "Turn On Indicator"=w242) -> ("Success?"=w238:bool)  [unwired: 6 in]
          }
          frame #1 {
            # "Start Digitizer"
            n123 = flat-sequence {
              tunnel: [w246] -> w245
              tunnel: w245 -> [w251]
              tunnel: [w251] -> w244
              frame #0 {
                n124 = control-ref of="Digitizer On"() -> (w249:refnum<vi>)
                n125 = control-ref of="Start Digi"() -> (w248:refnum<vi>)
                n126 = call "SwitchTillOn.vi"("Stop if On?"=FALSE, "timeout"=u32 5000, "Turn On Button"=w248, "Turn On Indicator"=w249) -> ("Success?"=w246:bool)  [unwired: 7 in]
              }
              frame #1 {
                n127 = local write "Digi Machine Mode"(T9."Scanning Mode" ("Digi Machine Mode")) -> ()
              }
              frame #2 {
                n128 = while {
                  stop <- w253 stop-if-true
                  n129 = local read "Digi Machine Mode"() -> (w255:T9)
                  n130 = Equal?(x=w255, y=T9."Scanning Mode") -> (x = y?=w253:bool)
                }
              }
            }
          }
          frame #2 {
            n131 = flat-sequence {
              frame #0 {
                n132 = while {
                  stop <- w259 stop-if-true
                  n133 = local read "Image State"() -> (w262:T7)
                  n134 = local read "Image State"() -> (w260:T7)
                  n135 = local write "Reset Img Ma"(TRUE ("Done Recording")) -> ()
                  n136 = Equal?(x=w260, y=PixelImageState."Update Pixel") -> (x = y?=w258:bool)
                  n137 = Equal?(x=w262, y=PixelImageState."Idle") -> (x = y?=w261:bool)
                  n138 = Or(x=w261, y=w258) -> (x .or. y?=w259:bool)
                }
                n139 = while {
                  stop <- w265 stop-if-true
                  n140 = local read "FileStore State"() -> (w269:T5)
                  n141 = local read "FileStore State"() -> (w267:T5)
                  n142 = local write "Done Recording"(TRUE ("Done Recording")) -> ()
                  n143 = Equal?(x=w267, y=Data_Save_State."Close File" ("FileStore State")) -> (x = y?=w264:bool)
                  n144 = Equal?(x=w269, y=Data_Save_State."Idle" ("FileStore State")) -> (x = y?=w268:bool)
                  n145 = Or(x=w268, y=w264) -> (x .or. y?=w265:bool)
                }
              }
              frame #1 {
                w272 = FALSE ("Done Recording")
                n146 = local write "Done Recording"(w272) -> ()
                n147 = local write "Reset Img Ma"(w272) -> ()
              }
            }
          }
          frame #3 {
            w273 = T10 {"Wave Count"=0, "Wave"=[]} ("input cluster")
            # "Flush All Queue"
            n148 = Obtain Queue(name (unnamed)="AquiredDataFIFOCopy", element data type=w273, create if not found? (T)=TRUE) -> (queue out=w279:refnum<queue>, error out=w277:errorcluster)  [unwired: 2 in, 1 out]
            n149 = Obtain Queue(name (unnamed)="AquiredDataFIFO", element data type=w273, create if not found? (T)=TRUE, error in (no error)=w277) -> (queue out=w280:refnum<queue>, error out=w278:errorcluster)  [unwired: 1 in, 1 out]
            n150 = while {
              tunnel: w280 -> [w296]
              tunnel: w279 -> [w295]
              shift-right: [w290] -> w276
              shift-left: w278 -> [w292]
              stop <- w285 stop-if-true
              n151 = Flush Queue(queue=w296, error in (no error)=w292) -> (queue out=w291:refnum<queue>, error out=w293:errorcluster)  [unwired: 1 out]
              n152 = Get Queue Status(queue=w291) -> (# elements in queue=w287:i32)  [unwired: 2 in, 7 out]
              n153 = Flush Queue(queue=w295, error in (no error)=w293) -> (queue out=w289:refnum<queue>, error out=w294:errorcluster)  [unwired: 1 out]
              n154 = Get Queue Status(queue=w289, error in (no error)=w294) -> (error out=w290:errorcluster, # elements in queue=w288:i32)  [unwired: 1 in, 6 out]
              n155 = Add(x=w288, y=w287) -> (x+y=w286:i32)
              n156 = Equal To 0?(x=w286) -> (x = 0?=w285:bool)
            }
            n157 = Unbundle By Name(w276) -> ("status"=w275:bool)
            n158 = Not(x=w275) -> (.not. x?=w274:bool)
          }
          frame #4 {
            # "Open File"
            n159 = case shown="True" "Save to File" {
              tunnel: [TRUE ("Success?") w302] -> w297
              frame False {
              }
              frame True {
                n160 = control-ref of="Done Recording"() -> (w300:refnum<vi>)
                n161 = control-ref of="File Open?"() -> (w303:refnum<vi>)
                n162 = control-ref of="Open File"() -> (w304:refnum<vi>)
                n163 = call "SwitchTillOn.vi"("Stop if On?"=TRUE, "Turn Off Button"=w300, "timeout"=u32 5000, "Turn On Button"=w304, "Turn On Indicator"=w303) -> ("Success?"=w302:bool)  [unwired: 6 in]
                n164 = local write "Record Data"(w302) -> ()
              }
            }
          }
          frame #5 {
            n165 = control-ref of="CountReset"() -> (w307:refnum<vi>)
            n166 = control-ref of="Wave Count Zero"() -> (w308:refnum<vi>)
            n167 = call "SwitchTillOn.vi"("Stop if On?"=FALSE, "timeout"=u32 5000, "Turn On Button"=w307, "Turn On Indicator"=w308) -> ("Success?"=w306:bool)  [unwired: 7 in]
          }
          frame #6 {
            w332 = 0.0 ("element")
            w341 = 1.0  # Offset
            # "Draw Markers To Indicate the Scan Area"
            n168 = property on="X End" class="DigNum (strict)"() -> ("Value"=w340:sgl)  [unwired: 2 in, 2 out]
            n169 = property on="X Start" class="DigNum (strict)"() -> ("Value"=w339:sgl)  [unwired: 2 in, 2 out]
            n170 = property on="Y End" class="DigNum (strict)"() -> ("Value"=w336:sgl)  [unwired: 2 in, 2 out]
            n171 = property on="Y Start" class="DigNum (strict)"() -> ("Value"=w338:sgl)  [unwired: 2 in, 2 out]
            n172 = Add(x=w341, y=w340) -> (x+y=w343:dbl)
            n173 = Subtract(x=w339, y=w341) -> (x-y=w344:dbl)
            n174 = Add(x=w336, y=w341) -> (x+y=w342:dbl)
            n175 = Subtract(x=w338, y=w341) -> (x-y=w337:dbl)
            n176 = Build Array(w339, w340) -> (w346:sgl[])
            n177 = Build Array(w338, w336) -> (w345:sgl[])
            n178 = property on="Stage Position" class="XYGraph (strict)"(error in=w335, "XScale.Maximum"=w343, "XScale.Minimum"=w344, "YScale.Maximum"=w342, "YScale.Minimum"=w337, "XScale.MarkerVals[]"=w346, "YScale.MarkerVals[]"=w345) -> (error out=w321:errorcluster)  [unwired: 1 in, 1 out]
            n179 = local read "EdgePt/nPixelMap"() -> (w325:bool)
            n180 = local read "IDs"() -> (w328:i32[])
            n181 = local read "Step Sizes"() -> (w326:sgl[])
            n182 = local read "Calibration"() -> (w327:cluster{dbl, "MicrostepMode":u32}[])
            n183 = call "SetSyncSettings.vi"("Periodic/nPointScan"=w325, "X SyncOut Enabled"=FALSE, "Y SyncOut Enabled"=FALSE, "error in (no error)"=w321, "Calibration"=w327, "Step Sizes(mm)"=w326, "IDs"=w328) -> ("error out"=w322:errorcluster)  [unwired: 3 in, 1 out]
            n184 = local read "IDs"() -> (w330:i32[])
            n185 = local read "Calibration"() -> (w331:cluster{dbl, "MicrostepMode":u32}[])
            n186 = local write "Next Coordinate Index"(0 ("Next Coordinate Index")) -> ()
            n187 = Build Array(w332, w332) -> (w333:dbl[])
            n188 = Compound Arithmetic op=AND(w316, w315, w314, w313, w311) -> (w312:bool)
            n189 = call "PositionControlRelative.vi"("Mode"=PosCtrlOptions."Both X and Y", "error in (no error)"=w322, "Calibration"=w331, "Move to"=w333, "IDs"=w330) -> ("error out"=w329:errorcluster)  [unwired: 4 in, 2 out]
            n190 = Select(t=StageOptions."Scan_Get Pos", s=w312, f=StageOptions."Idle") -> (s? t:f=w318:T3)
            n191 = local write "Scan Started"(w312) -> ()
          }
        }
        n192 = call <vilib>:"Unset Busy.vi"("error in (no error)"=w237) -> ("error out"=w233:errorcluster)  [unwired: 10 in]
      }
      frame "Scan_Get Pos" {
        n193 = local read "IDs"() -> (w360:i32[])
        n194 = local read "Calibration"() -> (w361:cluster{dbl, "MicrostepMode":u32}[])
        n195 = call "PositionControl.vi"("Mode"=PosCtrlOptions."Read Pos", "error in (no error)"=w363, "Calibration"=w361, "IDs"=w360) -> ("error out"=w362:errorcluster, "Moving?"=w352:bool, "Position"=w355:sgl[])  [unwired: 4 in, 1 out]
        n196 = local write "Moving?"(w352) -> ()
        n197 = Index Array(array=w355, index #1=0 ("index"), index #2=1 ("index")) -> (element #1=w349:sgl, element #2=w348:sgl)
        n198 = local write "X Position"(w349) -> ()
        n199 = local write "Y Position"(w348) -> ()
        n200 = Build Array(w349) -> (w358:sgl[])
        n201 = Build Array(w348) -> (w359:sgl[])
        n202 = Bundle(w358, w359) -> (w354:cluster{sgl[], sgl[]})  [unwired: 1 in]
        n203 = local write "Stage Position"(w354) -> ()
        n204 = property on="Stage Position" class="XYGraph (strict)"("Cursor.Cursor X"=w349, "Cursor.Cursor Y"=w348) -> ()  [unwired: 2 in, 2 out]
        n205 = Select(t=StageOptions."Scan_Get Pos", s=w352, f=StageOptions."Scan_SyncSet") -> (s? t:f=w353:T3)
      }
      frame "Scan_SyncSet" {
        n206 = local read "EdgePt/nPixelMap"() -> (w367:bool)
        n207 = local read "IDs"() -> (w375:i32[])
        n208 = local read "Step Sizes"() -> (w373:sgl[])
        n209 = local read "Calibration"() -> (w374:cluster{dbl, "MicrostepMode":u32}[])
        n210 = Quotient & Remainder(x="Next Coordinate Index", y=2) -> (x-y*floor(x/y)=w370:i32)  [unwired: 1 out]
        n211 = Not Equal To 0?(x=w370) -> (x != 0?=w368:bool)
        n212 = Compound Arithmetic op=OR(invert w367, w368) -> (w369:bool)
        n213 = call "SetSyncSettings.vi"("Periodic/nPointScan"=w367, "X SyncOut Enabled"=w369, "Y SyncOut Enabled"=FALSE, "error in (no error)"=w378, "Calibration"=w374, "Step Sizes(mm)"=w373, "IDs"=w375) -> ("error out"=w377:errorcluster)  [unwired: 3 in, 1 out]
      }
      frame "Scan_MoveNext" {
        n214 = flat-sequence {
          tunnel: w392 -> [w395]
          tunnel: [w395] -> w384
          tunnel: [w394] -> w383
          tunnel: [w393] -> w381
          tunnel: [w403] -> w390
          tunnel: [w400] -> w389
          tunnel: [w399] -> w385
          tunnel: w384 -> [w404]
          tunnel: w383 -> [w399]
          tunnel: [w398] -> w382
          tunnel: w381 -> [w398]
          tunnel: [w414] -> w380
          tunnel: [w415] -> w391
          tunnel: w382 -> [w407]
          tunnel: w385 -> [w411]
          tunnel: w389 -> [w412]
          tunnel: w390 -> [w415]
          frame #0 {
            n215 = local read "Machine Mode"() -> (w393:T8)
            n216 = case shown="\"Perimeter Mode\"" w393 {
              tunnel: [w396 w397] -> w394
              frame "Scanning Mode", Default {
                n217 = local read "Coordinate Array"() -> (w396:sgl[][])
              }
              frame "Perimeter Mode" {
                n218 = local read "Peripheral Coordis"() -> (w397:sgl[][])
              }
            }
          }
          frame #1 {
            n219 = local read "IDs"() -> (w402:i32[])
            n220 = local read "Calibration"() -> (w401:cluster{dbl, "MicrostepMode":u32}[])
            n221 = local read "Next Coordinate Index"() -> (w400:i32)
            n222 = Index Array(array=w399, index (row)=w400) -> (element=w405:sgl[])  [unwired: 1 in]
            n223 = call "PositionControl.vi"("Mode"=PosCtrlOptions."Both X and Y", "error in (no error)"=w404, "Calibration"=w401, "Move to"=w405, "IDs"=w402) -> ("error out"=w403:errorcluster)  [unwired: 3 in, 3 out]
          }
          frame #2 {
            n224 = Increment(x=w412) -> (x+1=w408:i32)
            n225 = Matrix Size(0:w411) -> (1:w410:i32)  [unwired: 1 out]
            n226 = Greater?(x=w408, y=w410) -> (0:w409:bool)
            n227 = case shown="True" w409 {
              selector: w409 -> [w416 _]
              tunnel: w408 -> [w417 w420]
              tunnel: [w417 w419] -> w413
              tunnel: [w416 w418] -> w414
              tunnel: w407 -> [_ w421]
              frame False {
              }
              frame True {
                n228 = case shown="\"Scanning Mode\", Default" w421 {
                  tunnel: w420 -> [w423 _]
                  tunnel: [w423 0] -> w419
                  tunnel: [TRUE ("x > y?") w425] -> w418
                  frame "Scanning Mode", Default {
                  }
                  frame "Perimeter Mode" {
                    n229 = local read "Outline"() -> (w426:bool)
                    n230 = Not(x=w426) -> (.not. x?=w425:bool)
                  }
                }
              }
            }
            n231 = local write "Next Coordinate Index"(w413) -> ()
          }
        }
        n232 = Not(x=w380) -> (.not. x?=w379:bool)
        n233 = Select(t=StageOptions."Scan_Complete", s=w380, f=StageOptions."Scan_Get Pos") -> (s? t:f=w388:T3)
      }
      frame "Scan_Complete" {
        n234 = stacked-sequence {
          tunnel: [w445 _] -> w431
          tunnel: w429 -> [w437 _]
          frame #0 {
            w434 = FALSE ("Y SyncOut Enabled")
            w443 = 0.0 ("element")
            # "Trigger After Reaching Zero to compensate For a Missed Trigger (If There)"
            n235 = local read "IDs"() -> (w440:i32[])
            n236 = local read "Step Sizes"() -> (w438:sgl[])
            n237 = local read "Calibration"() -> (w439:cluster{dbl, "MicrostepMode":u32}[])
            n238 = call "SetSyncSettings.vi"("Periodic/nPointScan"=w434, "X SyncOut Enabled"=TRUE, "Y SyncOut Enabled"=w434, "error in (no error)"=w437, "Calibration"=w439, "Step Sizes(mm)"=w438, "IDs"=w440) -> ("error out"=w436:errorcluster)  [unwired: 3 in, 1 out]
            n239 = local write "Scan Started"(FALSE ("Scan Started")) -> ()
            n240 = local write "Machine Mode"(T8."Normal" ("Machine Mode")) -> ()
            n241 = local read "IDs"() -> (w441:i32[])
            n242 = local read "Calibration"() -> (w442:cluster{dbl, "MicrostepMode":u32}[])
            n243 = Build Array(w443, w443) -> (w444:dbl[])
            n244 = call "PositionControl.vi"("Mode"=PosCtrlOptions."Both X and Y", "error in (no error)"=w436, "Calibration"=w442, "Move to"=w444, "IDs"=w441) -> ("error out"=w445:errorcluster)  [unwired: 3 in, 3 out]
          }
          frame #1 {
            n245 = local write "Digi Machine Mode"(T9."Single Shot Mode" ("y")) -> ()
          }
        }
      }
      frame "Cmd_MoveAbs" {
        n246 = local read "IDs"() -> (w453:i32[])
        n247 = local read "Calibration"() -> (w452:cluster{dbl, "MicrostepMode":u32}[])
        n248 = Build Array("X Position Abs", "Y Position Abs") -> (w451:dbl[])
        n249 = call "PositionControl.vi"("Mode"=PosCtrlOptions."Both X and Y", "error in (no error)"=w455, "Calibration"=w452, "Move to"=w451, "IDs"=w453) -> ("error out"=w454:errorcluster)  [unwired: 3 in, 3 out]
      }
      frame "Cmd_MoveStart" {
        n250 = local read "X Start"() -> (w458:sgl)
        n251 = local read "Y Start"() -> (w457:sgl)
        n252 = local read "IDs"() -> (w462:i32[])
        n253 = local read "Calibration"() -> (w461:cluster{dbl, "MicrostepMode":u32}[])
        n254 = Build Array(w458, w457) -> (w460:sgl[])
        n255 = call "PositionControl.vi"("Mode"=PosCtrlOptions."Both X and Y", "error in (no error)"=w464, "Calibration"=w461, "Move to"=w460, "IDs"=w462) -> ("error out"=w463:errorcluster)  [unwired: 3 in, 3 out]
      }
      frame "Cmd_CloseControllers" {
        n256 = local read "IDs"() -> (w467:i32[])
        n257 = for {
          shift-right: [w474] -> w471
          shift-left: w469 -> [w473]
          tunnel: w467 -> [w472] mode=indexing
          n258 = call "command stop.vi"("error in (no error)"=w473, "id"=w472) -> ("error out"=w474:errorcluster)  [unwired: 8 in, 1 out]
        }
        n259 = call "CloseDevices.vi"("error in (no error)"=w471, "Close"=TRUE, "Ids"=w467) -> ("error out"=w470:errorcluster)  [unwired: 8 in]
      }
      frame "Cmd_MoveUp" {
        n260 = local read "Move Step"() -> (w478:dbl)
        n261 = local read "IDs"() -> (w477:i32[])
        n262 = local read "Calibration"() -> (w476:cluster{dbl, "MicrostepMode":u32}[])
        n263 = Build Array(0.0 ("element"), w478) -> (w480:dbl[])
        n264 = call "PositionControlRelative.vi"("Mode"=PosCtrlOptions."Move Y", "error in (no error)"=w482, "Calibration"=w476, "Move to"=w480, "IDs"=w477) -> ("error out"=w481:errorcluster)  [unwired: 4 in, 2 out]
      }
      frame "Cmd_MoveDown" {
        n265 = local read "Move Step"() -> (w488:dbl)
        n266 = local read "IDs"() -> (w486:i32[])
        n267 = local read "Calibration"() -> (w485:cluster{dbl, "MicrostepMode":u32}[])
        n268 = Negate(x=w488) -> (-x=w487:dbl)
        n269 = Build Array(0.0 ("element"), w487) -> (w490:dbl[])
        n270 = call "PositionControlRelative.vi"("Mode"=PosCtrlOptions."Move Y", "error in (no error)"=w492, "Calibration"=w485, "Move to"=w490, "IDs"=w486) -> ("error out"=w491:errorcluster)  [unwired: 4 in, 2 out]
      }
      frame "Cmd_MoveLeft" {
        n271 = local read "Move Step"() -> (w499:dbl)
        n272 = local read "IDs"() -> (w495:i32[])
        n273 = local read "Calibration"() -> (w496:cluster{dbl, "MicrostepMode":u32}[])
        n274 = Negate(x=w499) -> (-x=w498:dbl)
        n275 = Build Array(w498, 0.0 ("element")) -> (w500:dbl[])
        n276 = call "PositionControlRelative.vi"("Mode"=PosCtrlOptions."Move X", "error in (no error)"=w502, "Calibration"=w496, "Move to"=w500, "IDs"=w495) -> ("error out"=w501:errorcluster)  [unwired: 4 in, 2 out]
      }
      frame "Cmd_MoveRight" {
        n277 = local read "Move Step"() -> (w508:dbl)
        n278 = local read "IDs"() -> (w506:i32[])
        n279 = local read "Calibration"() -> (w505:cluster{dbl, "MicrostepMode":u32}[])
        n280 = Build Array(w508, 0.0 ("element")) -> (w509:dbl[])
        n281 = call "PositionControlRelative.vi"("Mode"=PosCtrlOptions."Move X", "error in (no error)"=w511, "Calibration"=w505, "Move to"=w509, "IDs"=w506) -> ("error out"=w510:errorcluster)  [unwired: 4 in, 2 out]
      }
      frame "Cmd_MoveZero" {
        w516 = 0.0 ("element")
        n282 = local read "IDs"() -> (w514:i32[])
        n283 = local read "Calibration"() -> (w515:cluster{dbl, "MicrostepMode":u32}[])
        n284 = Build Array(w516, w516) -> (w517:dbl[])
        n285 = call "PositionControl.vi"("Mode"=PosCtrlOptions."Both X and Y", "error in (no error)"=w519, "Calibration"=w515, "Move to"=w517, "IDs"=w514) -> ("error out"=w518:errorcluster)  [unwired: 3 in, 3 out]
      }
      frame "Cmd_GetPos" {
        n286 = local read "IDs"() -> (w531:i32[])
        n287 = local read "Calibration"() -> (w532:cluster{dbl, "MicrostepMode":u32}[])
        n288 = call "PositionControl.vi"("Mode"=PosCtrlOptions."Read Pos", "error in (no error)"=w534, "Calibration"=w532, "IDs"=w531) -> ("error out"=w533:errorcluster, "Moving?"=→"Moving?":bool, "Position"=w525:sgl[])  [unwired: 4 in, 1 out]
        n289 = Index Array(array=w525, index #1=0 ("index"), index #2=1 ("index")) -> (element #1=w522:sgl, element #2=w521:sgl)
        n290 = local write "X Position"(w522) -> ()
        n291 = local write "Y Position"(w521) -> ()
        n292 = Build Array(w522) -> (w529:sgl[])
        n293 = Build Array(w521) -> (w530:sgl[])
        n294 = Bundle(w529, w530) -> (→"Stage Position":cluster{sgl[], sgl[]})  [unwired: 1 in]
        n295 = property on="Stage Position" class="XYGraph (strict)"("Cursor.Cursor X"=w522, "Cursor.Cursor Y"=w521) -> ()  [unwired: 2 in, 2 out]
      }
      frame "Cmd_Stop" {
        n296 = local read "IDs"() -> (w537:i32[])
        n297 = for {
          shift-right: [w542] -> w539
          shift-left: w538 -> [w541]
          tunnel: w537 -> [w540] mode=indexing
          n298 = call "command stop.vi"("error in (no error)"=w541, "id"=w540) -> ("error out"=w542:errorcluster)  [unwired: 8 in, 1 out]
        }
      }
      frame "Sync_On" {
        n299 = local read "EdgePt/nPixelMap"() -> (w545:bool)
        n300 = local read "IDs"() -> (w548:i32[])
        n301 = local read "Step Sizes"() -> (w546:sgl[])
        n302 = local read "Calibration"() -> (w547:cluster{dbl, "MicrostepMode":u32}[])
        n303 = call "SetSyncSettings.vi"("Periodic/nPointScan"=w545, "X SyncOut Enabled"=TRUE, "Y SyncOut Enabled"=FALSE, "error in (no error)"=w551, "Calibration"=w547, "Step Sizes(mm)"=w546, "IDs"=w548) -> ("error out"=w550:errorcluster)  [unwired: 3 in, 1 out]
      }
      frame "Sync_Off" {
        n304 = local read "EdgePt/nPixelMap"() -> (w554:bool)
        n305 = local read "IDs"() -> (w557:i32[])
        n306 = local read "Step Sizes"() -> (w555:sgl[])
        n307 = local read "Calibration"() -> (w556:cluster{dbl, "MicrostepMode":u32}[])
        n308 = call "SetSyncSettings.vi"("Periodic/nPointScan"=w554, "X SyncOut Enabled"=FALSE, "Y SyncOut Enabled"=FALSE, "error in (no error)"=w560, "Calibration"=w556, "Step Sizes(mm)"=w555, "IDs"=w557) -> ("error out"=w559:errorcluster)  [unwired: 3 in, 1 out]
      }
      frame "Stop Motion" {
        w563 = TRUE ("Close")
        n309 = local read "IDs"() -> (w565:i32[])
        n310 = for {
          shift-right: [w571] -> w568
          shift-left: w566 -> [w570]
          tunnel: w565 -> [w569] mode=indexing
          n311 = call "command stop.vi"("error in (no error)"=w570, "id"=w569) -> ("error out"=w571:errorcluster)  [unwired: 8 in, 1 out]
        }
        n312 = call "CloseDevices.vi"("error in (no error)"=w568, "Close"=w563, "Ids"=w565) -> ("error out"=w567:errorcluster)  [unwired: 8 in]
        n313 = local write "Moving?"(FALSE ("Moving?")) -> ()
        n314 = local write "Machine Mode"(T8."Normal" ("Machine Mode")) -> ()
      }
      frame "CloseApplication" {
        w573 = TRUE ("Close")
        n315 = local read "IDs"() -> (w576:i32[])
        n316 = local write "Moving?"(FALSE ("Moving?")) -> ()
        n317 = for {
          shift-right: [w582] -> w579
          shift-left: w577 -> [w581]
          tunnel: w576 -> [w580] mode=indexing
          n318 = call "command stop.vi"("error in (no error)"=w581, "id"=w580) -> ("error out"=w582:errorcluster)  [unwired: 8 in, 1 out]
        }
        n319 = call "CloseDevices.vi"("error in (no error)"=w579, "Close"=w573, "Ids"=w576) -> ("error out"=w578:errorcluster)  [unwired: 8 in]
        n320 = local write "Machine Mode"(T8."Normal" ("Machine Mode")) -> ()
      }
    }
    "Scan Running" <- w45
    n321 = local read "Serial nos"() -> (w51:u32[])
    n322 = call <instrlib>:"Synchronous Latch.vi"("clear"=w59, "set"=w61) -> ("out"=w60:bool)  [unwired: 9 in]
    n323 = call <instrlib>:"Synchronous Latch.vi"("clear"=w46, "set"=w48) -> ("out"=→"Scan Complete":bool)  [unwired: 9 in]
    n324 = Not(x=w60) -> (.not. x?=w53:bool)
    n325 = Greater Than 0?(x=w51) -> (x > 0?=w50:bool[])
    n326 = Or(x=w65, y="Stop Stage") -> (x .or. y?=w62:bool)
    n327 = And Array Elements(Boolean array=w50) -> (logical AND=w49:bool)
    n328 = Select(t=StageOptions."Stop Motion", s=w62, f=w63) -> (s? t:f=w56:T3)
    n329 = And(x=w49, y=w53) -> (x .and. y?=→"Controller Open?":bool)
    n330 = Select(t=StageOptions."CloseApplication", s="Stop Stage App", f=w56) -> (s? t:f=w57:T3)
    "Stage Status" <- w68
  }
  n331 = timed-loop "Generator Control" {
    shift-right: [w591] -> _
    shift-left: Generator_States."Idle" -> [w594]
    shift-right: [w592] -> w6
    shift-left: errorcluster {"status"=FALSE, "code"=0, "source"=""} ("error in") -> [w593]
    timing: w36 -> [_]
    timing-out: [_] -> w35
    stop <- w583 stop-if-true
    n332 = node-c288() -> ()  [unwired: 1 in, 1 out]
    n333 = case shown="\"Idle\", Default" w594 {
      tunnel: [w597 Generator_States."InitGen" Generator_States."Idle" Generator_States."Idle" Generator_States."Idle" Generator_States."Idle"] -> w590
      tunnel: w593 -> [w605 w618 w631 w637 w642 w647]
      tunnel: [w605 w612 w622 w636 w641 w646] -> w592
      tunnel: [_ _ TRUE ("Ext/nViTrig") _ _ _] -> w588
      tunnel: [w604 _ _ _ TRUE ("x .or. y?") w643] -> w587
      tunnel: [_ _ _ _ _ w643] -> w583
      frame "Idle", Default {
        n334 = Build Array("Send vi Trig", "Start Gen", "stop Gen", FALSE ("element")) -> (w603:bool[])
        n335 = Boolean Array To Number(Boolean array=w603) -> (number=w598:u32)
        n336 = case shown="4" w598 {
          tunnel: [Generator_States."Idle" ("f") Generator_States."SendVITrig" Generator_States."GenerateWaveArray" Generator_States."CloseGen"] -> w597
          frame 0, Default {
          }
          frame 1 {
          }
          frame 2 {
          }
          frame 4 {
          }
        }
        n337 = First Call?() -> (First Call?: T/F=w604:bool)
      }
      frame "GenerateWaveArray" {
        n338 = call "WaveSynthV2.vi"("error in"=w618, "Default Wave"="Use Default Wave Settings") -> ("error out"=w612:errorcluster, "Waves per Pixel"=→"Waves per Pixel":u32, "Sampling Frequency (Hz)"=→"Sampling Frequency (Hz)":u64, "Amplitudes"=→"Amplitudes" →"Input Waveform":dbl[], "Offset Factor"=→"Offset Factor":dbl, "Gain"=→"Gain":dbl)  [unwired: 2 in]
      }
      frame "InitGen" {
        n339 = local read "Gain"() -> (w626:dbl)
        n340 = local read "Amplitudes"() -> (w627:dbl[])
        n341 = local read "Sampling Frequency (Hz)"() -> (w629:u64)
        n342 = local read "Waves per Pixel"() -> (w628:u32)
        n343 = local read "Offset Factor"() -> (w625:dbl)
        n344 = call "InitGen.vi"("Offset"=w625, "Gain"=w626, "Ext/nViTrig"="Ext/nViTrig", "Waveform Data Array"=w627, "error in (no error)"=w631, "Wave Per Pixel"=w628, "Sample Rate (Samp/s)"=w629, "FGEN Resource Name"="Generator  Port") -> ("error out"=w623:errorcluster, "Actual Sample Rate"=→"Actual Sample Rate":dbl, "reference out"=w621:refnum<k15>)  [unwired: 1 in]
        n345 = call "EnableOutput.vi"("error in (no error)"=w623, "FGEN Resource Name"=w621) -> ("error out"=w622:errorcluster)  [unwired: 8 in, 1 out]
      }
      frame "SendVITrig" {
        n346 = local read "Generator  Port"() -> (w634:refnum<k15>)
        n347 = call "SendTrig.vi"("error in (no error)"=w637, "Send vi Trig"=TRUE, "Instrument Handle"=w634) -> ("error out"=w636:errorcluster)  [unwired: 7 in, 1 out]
      }
      frame "CloseGen" {
        n348 = local read "Generator  Port"() -> (w640:refnum<k15>)
        n349 = call "CloseGen.vi"("error in (no error)"=w642, "Instrument Handle"=w640) -> ("error out"=w641:errorcluster)  [unwired: 9 in]
      }
      frame "CloseApp" {
        w643 = TRUE ("x .or. y?")
        n350 = local read "Generator  Port"() -> (w645:refnum<k15>)
        n351 = call "CloseGen.vi"("error in (no error)"=w647, "Instrument Handle"=w645) -> ("error out"=w646:errorcluster)  [unwired: 9 in]
      }
    }
    n352 = call <instrlib>:"Synchronous Latch.vi"("clear"=w587, "set"=w588) -> ("out"=→"Generator On":bool)  [unwired: 9 in]
    n353 = Or(x="Stop Gen App", y=w592) -> (x .or. y?=w584:bool)
    n354 = node-c288() -> ()  [unwired: 1 in, 1 out]
    n355 = Select(t=Generator_States."CloseApp", s=w584, f=w590) -> (s? t:f=w591:T6)
    "Gen State" <- w594
  }
  "Error Out Gen" <- w6
  n356 = while {
    stop <- w648 stop-if-true
    n357 = event shown="[1] \"EXIT APP\": Value Change" {
      selector: _ -> [_ _]
      dyn-events: _ -> [_ _]
      timeout: _ -> [_ _]
      tunnel: [_ w652] -> w648
      event Timeout {
        n358 = event-data() -> ()  [unwired: 1 in, 3 out]
      }
      event "EXIT APP": Value Change {
        n359 = event-data() -> ()  [unwired: 1 in, 6 out]
        n360 = flat-sequence {
          tunnel: [w653] -> w651
          tunnel: w651 -> [w656]
          tunnel: [w655] -> w650
          tunnel: w650 -> [w670]
          tunnel: [w669] -> w649
          tunnel: w649 -> [w672]
          tunnel: ["EXIT APP"] -> w652
          frame #0 {
            w654 = TRUE ("Stop Gen App")
            n361 = local write "Stop Stage App"(w654) -> ()
            n362 = local write "Stop Gen App"(w654) -> ()
            n363 = local write "Stop Digi App"(w654) -> ()
            n364 = local write "Stop File App"(w654) -> ()
            n365 = Tick Count (ms)() -> (millisecond timer value=w653:u32)
          }
          frame #1 {
            n366 = while {
              shift-right: [w663] -> _
              shift-left: w656 -> [w663]
              tunnel: [w657] -> w655
              stop <- w660 stop-if-true
              n367 = local read "Generator On"() -> (w668:bool)
              n368 = local read "File Open?"() -> (w667:bool)
              n369 = local read "Digitizer On"() -> (w666:bool)
              n370 = local read "Controller Open?"() -> (w665:bool)
              n371 = Tick Count (ms)() -> (millisecond timer value=w664:u32)
              n372 = Subtract(x=w664, y=w663) -> (x-y=w662:u32)
              n373 = Greater?(x=w662, y=u32 5000) -> (0:w659:bool)
              n374 = Compound Arithmetic op=OR(w668, w667, w666, w665) -> (invert w658:bool)
              n375 = Or(x=w658, y=w659) -> (x .or. y?=w660:bool)
              n376 = Not(x=w658) -> (.not. x?=w657:bool)
            }
          }
          frame #2 {
            w671 = FALSE ("Stop Gen App")
            n377 = call "Display Message to User"("Enable"=w670) -> ("error out"=w669:errorcluster)  [unwired: 9 in, 1 out]
            n378 = local write "Stop Stage App"(w671) -> ()
            n379 = local write "Stop Gen App"(w671) -> ()
            n380 = local write "Stop Digi App"(w671) -> ()
            n381 = local write "Stop File App"(w671) -> ()
          }
          frame #3 {
            w675 = TRUE ("force destroy? (F)")
            n382 = Obtain Queue(name (unnamed)="AquiredDataFIFOCopy", element data type=T10 {"Wave Count"=0, "Wave"=[]} ("input cluster"), create if not found? (T)=TRUE, error in (no error)=w672) -> (queue out=w677:refnum<queue>, error out=w673:errorcluster)  [unwired: 1 in, 1 out]
            n383 = Obtain Queue(name (unnamed)="AquiredDataFIFO", element data type=T10 {"Wave Count"=0, "Wave"=[]} ("input cluster"), create if not found? (T)=TRUE, error in (no error)=w673) -> (queue out=w678:refnum<queue>, error out=w674:errorcluster)  [unwired: 1 in, 1 out]
            n384 = Release Queue(queue=w678, force destroy? (F)=w675, error in (no error)=w674) -> (error out=w676:errorcluster)  [unwired: 2 out]
            n385 = Release Queue(queue=w677, force destroy? (F)=w675, error in (no error)=w676) -> ()  [unwired: 3 out]
          }
          frame #4 {
            n386 = Stop(stop? (T)="EXIT APP") -> ()
          }
        }
      }
    }
  }
  n387 = timed-loop {
    timing: w5 -> [_]
    timing-out: [_] -> w4
    stop <- _ stop-if-true
    n388 = node-c288() -> ()  [unwired: 1 in, 1 out]
    n389 = event shown="[2] \"LIVE\": Value Change" {
      selector: _ -> [_ _ _ _ _ _]
      dyn-events: _ -> [_ _ _ _ _ _]
      timeout: 0 -> [_ _ _ _ _ _]
      event Timeout {
        w687 = FALSE ("Start Digi")
        n390 = event-data() -> ()  [unwired: 1 in, 3 out]
        n391 = local read "Digi Machine Mode"() -> (w688:T9)
        n392 = local write "Trigger Digi Single"(w687) -> ()
        n393 = local write "Start Digi"(w687) -> ()
        n394 = case shown="\"Scanning Mode\"" w688 {
          frame "Live Mode" {
            w689 = FALSE ("Value (Signaling)")
            n395 = Not(x=w689) -> (.not. x?=w690:bool)
            n396 = local write "Single Shot"(w689) -> ()
            n397 = local write "Scanning"(w689) -> ()
            n398 = local write "LIVE"(w690) -> ()
          }
          frame "Single Shot Mode" {
            w692 = FALSE ("Value (Signaling)")
            n399 = Not(x=w692) -> (.not. x?=w691:bool)
            n400 = local write "Single Shot"(w691) -> ()
            n401 = local write "Scanning"(w692) -> ()
            n402 = local write "LIVE"(w692) -> ()
          }
          frame "Scanning Mode" {
            w694 = FALSE ("Value (Signaling)")
            n403 = Not(x=w694) -> (.not. x?=w693:bool)
            n404 = local write "Single Shot"(w694) -> ()
            n405 = local write "Scanning"(w693) -> ()
            n406 = local write "LIVE"(w694) -> ()
          }
        }
      }
      event "TriggerDigi": Value Change {
        n407 = event-data() -> ()  [unwired: 1 in, 6 out]
        n408 = local write "Trigger Digi Single"(TRUE ("Trigger Digi Single")) -> ()
      }
      event "LIVE": Value Change {
        n409 = event-data() -> ()  [unwired: 1 in, 6 out]
        n410 = local write "Digi Machine Mode"(T9."Live Mode" ("Digi Machine Mode")) -> ()
      }
      event "Single Shot": Value Change {
        n411 = event-data() -> ()  [unwired: 1 in, 6 out]
        n412 = local write "Digi Machine Mode"(T9."Single Shot Mode" ("Digi Machine Mode")) -> ()
      }
      event "Scanning": Value Change {
        n413 = event-data() -> ()  [unwired: 1 in, 6 out]
        n414 = local write "Digi Machine Mode"(T9."Scanning Mode" ("Digi Machine Mode")) -> ()
      }
      event "Start Digitizer UI Bttn": Value Change {
        n415 = event-data() -> ()  [unwired: 1 in, 6 out]
        n416 = local write "Start Digi"(TRUE ("Start Digi")) -> ()
      }
    }
    n417 = node-c288() -> ()  [unwired: 1 in, 1 out]
  }
  n418 = node-c288(w4) -> ()  [unwired: 1 out]
  n419 = node-c288(w35) -> ()  [unwired: 1 out]
  n420 = Obtain Queue(name (unnamed)="AquiredDataFIFO", element data type=T10 {"Wave Count"=0, "Wave"=[]} ("input cluster"), create if not found? (T)=TRUE) -> (queue out=w25:refnum<queue>, error out=w24:errorcluster)  [unwired: 2 in, 1 out]
  n421 = Obtain Queue(name (unnamed)="AquiredDataFIFOCopy", element data type=T10 {"Wave Count"=0, "Wave"=[]} ("input cluster"), create if not found? (T)=TRUE) -> (queue out=w7:refnum<queue>, error out=w8:errorcluster)  [unwired: 2 in, 1 out]
  n422 = while "Signal View" {
    shift-right: [w726] -> _
    shift-left: dbl[][] [] -> [w725]
    shift-right: [w715] -> _
    shift-left: PixelImageState."Idle" -> [w727]
    shift-right: [w723] -> _
    shift-left: u32[][] [] -> [w724]
    shift-right: [w722] -> _
    shift-left: sgl[] [] -> [w721]
    shift-right: [w720] -> _
    shift-left: sgl[] [] -> [w719]
    shift-right: [w712] -> _
    shift-left: w25 -> [w713]
    shift-right: [w710] -> _
    shift-left: w24 -> [w711]
    tunnel: [w703] -> w1
    stop <- w702 stop-if-true
    n423 = call <extravilib>:"Read.vi"("channel"=w703) -> ("element"=w702:bool)  [unwired: 1 in, 1 out]
    n424 = Get Queue Status(queue=w713, error in (no error)=w711) -> (queue out=w712:refnum<queue>, error out=w710:errorcluster, # elements in queue=w709:i32)  [unwired: 1 in, 5 out]
    n425 = Greater Than 0?(x=w709) -> (x > 0?=w705:bool)
    n426 = case shown="True" w705 {
      tunnel: w712 -> [_ w750]
      tunnel: [_ w749] -> w708
      tunnel: [_ w748] -> w707
      tunnel: [_ w731] -> w706
      tunnel: [TRUE ("timed out?") w730] -> w704
      frame False {
      }
      frame True {
        n427 = Dequeue Element(queue=w750, timeout in ms (-1)=200) -> (element=w731:T10, timed out?=w730:bool)  [unwired: 1 in, 2 out]
        n428 = local read "Time Division"() -> (w746:u8)
        n429 = control-ref of="Waveform [LIVE]"() -> (w739:refnum<vi>)
        n430 = Unbundle By Name(w731) -> ("Wave"=w735:i16[])
        n431 = local read "Range (Vpp)"() -> (w740:dbl)
        n432 = local read "Delay(us)"() -> (w742:sgl)
        n433 = Power Of 2(x=w746) -> (2^x=w745:dbl)
        n434 = Divide(x=1600000000.0 ("Sample Rate"), y=w745) -> (x/y=w744:dbl)
        n435 = call "Scale Acquired Data.vi"("range (V)"=w740, "Start Time (us)"=w742, "Sample Rate"=w744, "Number of Bits"=i16 16, "Data In"=w735) -> ("output waveform"=w741:cluster{"Start Time":dbl, dbl, ext[]})  [unwired: 6 out]
        n436 = call "ShowMinMaxOn Graoh.vi"("Log Mode?"="LogMode", "WaveformGraph in"=w739, "Range (Vpp)"=w740, "output waveform"=w741) -> ("max index Log"=w749:i32, "Max Log"=w748:ext, "Time (sec)"=→"Max Index (s)":dbl, "Max Abs"=→"Max Val (V)":ext)  [unwired: 4 in]
        n437 = call-poly <instrlib>:"Count Up.vi"("increment"=TRUE, "reset"="reset Rx wave count") -> ("count out"=→"Waves Received":u32)  [unwired: 13 in]
      }
    }
    n438 = case shown="\"Update Pixel\"" w727 {
      tunnel: [w760 w775 w812 dbl[][] []] -> w726
      tunnel: w725 -> [_ w777 w812 _]
      tunnel: w708 -> [_ w772 _ _]
      tunnel: w707 -> [_ w776 _ _]
      tunnel: [PixelImageState."Update Pixel" w774 PixelImageState."Idle" ("f") w818] -> w714
      tunnel: w724 -> [_ w773 w810 _]
      tunnel: [w759 w769 w810 u32[][] []] -> w723
      tunnel: [w752 w766 _ _] -> w722
      tunnel: w721 -> [_ w771 _ _]
      tunnel: [w751 w765 _ _] -> w720
      tunnel: w719 -> [_ w770 _ _]
      tunnel: w706 -> [_ w768 _ _]
      tunnel: w704 -> [_ w767 _ _]
      frame "Init" {
        n439 = local read "Pixel Count"() -> (w755:i32)
        n440 = local read "Line Count"() -> (w756:i32)
        n441 = Initialize Array(0.0 ("element"), w756, w755) -> (w760:dbl[][])
        n442 = local read "Y Step Size (R)"() -> (w754:sgl)
        n443 = local read "X Step Size (R)"() -> (w753:sgl)
        n444 = for {
          N: w756 -> [_]
          tunnel: [w764] -> w757 mode=indexing
          i -> [w764]
        }
        n445 = for {
          N: w755 -> [_]
          tunnel: [w763] -> w758 mode=indexing
          i -> [w763]
        }
        n446 = Multiply(x=w757, y=w754) -> (x*y=w752:sgl[])
        n447 = Multiply(x=w758, y=w753) -> (x*y=w751:sgl[])
        n448 = To Unsigned Long Integer(number=w760) -> (unsigned 32bit integer=w759:u32[][])
      }
      frame "Update Pixel" {
        n449 = case shown="False" w767 {
          tunnel: w777 -> [w803 w805]
          tunnel: w776 -> [w802 _]
          tunnel: [w800 w805] -> w775
          tunnel: [w794 PixelImageState."Update Pixel" ("f")] -> w774
          tunnel: w773 -> [w789 w806]
          tunnel: w772 -> [w786 _]
          tunnel: w771 -> [w780 w808]
          tunnel: w770 -> [w779 w807]
          tunnel: [w783 w806] -> w769
          tunnel: w768 -> [w782 _]
          tunnel: [w780 w808] -> w766
          tunnel: [w779 w807] -> w765
          frame False {
            n450 = local read "PixelMap_Scan"() -> (w792:i32[][])
            n451 = Unbundle By Name(w782) -> ("Wave Count"=w781:u32)
            n452 = Index Array(array=w792, index (row)=w781) -> (element=w804:i32[])  [unwired: 1 in]
            n453 = Increment(x=w781) -> (x+1=w778:u32)
            n454 = Matrix Size(0:w792) -> (1:w791:i32)  [unwired: 1 out]
            n455 = Index Array(array=w804) -> (element #1=w787:i32, element #2=w788:i32)  [unwired: 2 in]
            n456 = Less?(x=w778, y=w791) -> (x < y?=w790:bool)
            n457 = Replace Array Subset(array=w803, new element=w802, index (row)=w788, index (col)=w787) -> (w800:dbl[][])
            n458 = control-ref of="Scanned Image"() -> (w795:refnum<vi>)
            n459 = call "DisplayImagePlot.vi"("Data Array"=w800, "Picture For Size Ref"=w795, "Colorbar"="ColorBar", "Axis"="Axis", "Map"="Map") -> ("Picture"=→"Scanned Image":picture)  [unwired: 6 in]
            n460 = Replace Array Subset(array=w789, new element=w786, index (row)=w788, index (col)=w787) -> (w783:u32[][])
            n461 = call <vilib>:"create_plot_surface.vi"("z matrix"=w783, "y vector"=w779, "x vector"=w780) -> ("plots out"=→"Topography Plot":refnum<class "Base Datatype.lvclass">[])  [unwired: 2 in, 6 out]
            n462 = property on="Topography Plot" class="LabVIEW 3D Graph (strict)"("property_graph_fast_draw"=TRUE ("Graph:Fast Draw")) -> ()  [unwired: 2 in, 2 out]
            n463 = Select(t=PixelImageState."Update Pixel", s=w790, f=PixelImageState."Complete Imaging") -> (s? t:f=w794:T7)
          }
          frame True {
          }
        }
      }
      frame "Complete Imaging" {
      }
      frame "Idle", Default {
        n464 = Select(t=PixelImageState."Init", s="Scan Started", f=PixelImageState."Idle") -> (s? t:f=w818:T7)
      }
    }
    n465 = call <instrlib>:"Detect Rising Edge.vi"("signal"="Reset Img Ma") -> ("edge detected"=w717:bool)  [unwired: 14 in]
    n466 = Select(t=PixelImageState."Idle", s=w717, f=w714) -> (s? t:f=w715:T7)
    "Image State" <- w727
  }
  n467 = while {
    shift-right: [w832] -> w15
    shift-left: w29 -> [w845]
    shift-right: [w844] -> _
    shift-left: _ -> [w843]
    shift-right: [w834] -> _
    shift-left: Digitizer_StatesMain."Idle" -> [w846]
    shift-right: [w840] -> _
    shift-left: w39 -> [w839]
    shift-right: [w830] -> _
    shift-left: w28 -> [w831]
    shift-right: [w828] -> _
    shift-left: w16 -> [w829]
    shift-right: [w826] -> _
    shift-left: w12 -> [w822]
    tunnel: w1 -> [w819]
    stop <- w820 stop-if-true
    n468 = Equal To 0?(x=w822) -> (x = 0?=→"Wave Count Zero":bool)
    n469 = case shown="\"VITrig\"" w846 {
      tunnel: w845 -> [w849 w879 w907 w924 w953 w972]
      tunnel: [w849 w860 w900 w923 w938 w970] -> w832
      tunnel: [w854 w871 w890 w918 w943 _] -> w844
      tunnel: w843 -> [w854 _ w892 w919 w946 w971]
      tunnel: [w855 Digitizer_StatesMain."SetParam" ("f") w896 Digitizer_StatesMain."Read" ("f") w948 Digitizer_StatesMain."Idle" ("f")] -> w833
      tunnel: [_ _ w898 _ _ _] -> w841
      tunnel: [w853 _ w894 w920 w947 _] -> w840
      tunnel: w839 -> [w853 _ _ w920 w947 _]
      tunnel: [TRUE _ _ _ _ w969] -> w838
      tunnel: [_ _ _ _ _ w969] -> w821
      tunnel: w831 -> [w850 w866 w886 w911 w937 w967]
      tunnel: [w850 w865 w886 w911 w936 w967] -> w830
      tunnel: [w848 w863 w885 w910 w933 w966] -> w828
      tunnel: w829 -> [w848 w862 w885 w910 w934 w966]
      tunnel: [u16 0 ("Wave Count") u16 0 ("Wave Count") w883 w908 w929 u16 0 ("Wave Count")] -> w827
      tunnel: w822 -> [_ _ w884 w908 w926 _]
      frame "Idle", Default {
        w851 = FALSE ("TIS Configured?")
        n470 = local write "TIS Configured?"(w851) -> ()
        n471 = local write "Configured?"(w851) -> ()
        n472 = Select(t=Digitizer_StatesMain."Init", s="Start Digi", f=Digitizer_StatesMain."Idle") -> (s? t:f=w855:T4)
      }
      frame "Init" {
        n473 = xnode "Open FPGA VI Reference"("error in"=w879, "resource name"="RIO Resource") -> ("FPGA VI Reference Out"=w869:refnum<k20>, "error out"=w878:errorcluster)
        n474 = Type Cast(type=T17 refnum ("FPGA VI Reference Out"), x=w869) -> (*(type *) &x=w868:T17)
        n475 = call "InitDigitizer.vi"("error in"=w878, "FPGA VI Reference In"=w868) -> ("error out"=w873:errorcluster, "range (Vpp)"=→"Range (Vpp)":dbl, "FPGA VI Reference Out"=w874:T17, "TIS Configured?"=→"TIS Configured?":bool, "Configured?"=→"Configured?":bool)  [unwired: 5 in]
        n476 = call "PXITrigReserve-Unreserve.vi"("error in"=w873, "Mode"=enum16{"Reserve", "Unreserve"}."Reserve", "FPGA VI Reference In"=w874) -> ("error out"=w864:errorcluster, "FPGA VI Reference Out"=w871:T17)  [unwired: 7 in]
        n477 = Flush Queue(queue=w866, error in (no error)=w864) -> (queue out=w865:refnum<queue>, error out=w861:errorcluster)  [unwired: 1 out]
        n478 = Flush Queue(queue=w862, error in (no error)=w861) -> (queue out=w863:refnum<queue>, error out=w860:errorcluster)  [unwired: 1 out]
      }
      frame "SetParam" {
        w904 = FALSE  # vi/nGenTrig
        w887 = sgl 5000.0  # ProcessCompletionDelay Factor
        # "Dis-Arm the trigger before seting the parameters! and then Arm Again"
        n479 = local read "Digi Machine Mode"() -> (w893:T9)
        n480 = call "ConfigAquisitionParam.vi"("Requested Samples Per Pixel"="Record Size", "Downsample [0,1,2]"="Time Division", "ProcessCompletionDelay (us)"=w887, "vi/nGenTrig"=w904, "error in"=w907, "AvgCount_powerOf2"="Amplitude \nAveraging", "Delay (us)"="Delay(us)", "FPGA VI Reference In"=w892) -> ("error out"=w902:errorcluster, "Read Size (Host)"=w894:u16, "FPGA VI Reference Out"=w891:T17)  [unwired: 1 in]
        n481 = Equal?(x=w893, y=T9."Scanning Mode") -> (x = y?=w882:bool)
        n482 = Select(t=Digitizer_StatesMain."Read" ("f"), s=w882, f=Digitizer_StatesMain."VITrig") -> (s? t:f=w896:T4)
        n483 = call "Arm(CommitSettings).vi"("Arm?"=TRUE, "error in"=w902, "FPGA VI Reference In"=w891) -> ("error out"=w900:errorcluster, "FPGA VI Reference Out"=w890:T17)  [unwired: 7 in]
        n484 = Unbundle By Name(w900) -> ("status"=w899:bool)
        n485 = Select(t=u16 0, s=w882, f=w884) -> (s? t:f=w883:u16)
        n486 = Not(x=w899) -> (.not. x?=w898:bool)
      }
      frame "VITrig" {
        n487 = Not(x="Pause Triggger") -> (.not. x?=w909:bool)
        n488 = call <instrlib>:"Detect Rising Edge.vi"("signal"="Trigger Digi Single") -> ("edge detected"=w913:bool)  [unwired: 14 in]
        n489 = Equal?(x="Digi Machine Mode", y=T9."Single Shot Mode") -> (x = y?=w915:bool)
        n490 = Select(t=w913, s=w915, f=w909) -> (s? t:f=w912:bool)
        n491 = call "ViTrig.vi"("Vi Trigger"=w912, "error in"=w924, "FPGA VI Reference In"=w919) -> ("error out"=w923:errorcluster, "FPGA VI Reference Out"=w918:T17)  [unwired: 7 in]
        n492 = case shown="True" w909 {
          frame False {
          }
          frame True {
            n493 = Wait (ms)(milliseconds to wait=u32 15) -> ()  [unwired: 1 out]
          }
        }
      }
      frame "Read" {
        n494 = call "ReadFromDigi.vi"("Timeout (ms)"=500, "error in"=w953, "Number of Elements"=w947, "FPGA VI Reference In"=w946) -> ("error out"=w942:errorcluster, "Data Valid?"=w928:bool, "Output Waveform"=w939:u16[], "FPGA VI Reference Out"=w944:T17)  [unwired: 4 in]
        n495 = To Word Integer(number=w939) -> (16bit integer=w932:i16[])
        n496 = Increment(x=w926) -> (x+1=w927:u16)
        n497 = Bundle By Name(cluster=T10 {"Wave Count"=0, "Wave"=[]} ("input cluster"), "Wave Count"=w926, "Wave"=w932) -> (w930:T10)
        n498 = Select(t=w927, s=w928, f=w926) -> (s? t:f=w929:u16)
        n499 = call "Arm(CommitSettings).vi"("Arm?"=TRUE, "error in"=w942, "FPGA VI Reference In"=w944) -> ("error out"=w935:errorcluster, "FPGA VI Reference Out"=w943:T17)  [unwired: 7 in]
        n500 = local read "Digi Machine Mode"() -> (w945:T9)
        n501 = case shown="True" w928 {
          tunnel: w930 -> [_ w960]
          tunnel: w935 -> [w956 w959]
          tunnel: [w956 w957] -> w938
          tunnel: w937 -> [w955 w964]
          tunnel: [w955 w963] -> w936
          tunnel: w934 -> [w954 w962]
          tunnel: [w954 w961] -> w933
          frame False {
          }
          frame True {
            n502 = Enqueue Element(queue=w964, element=w960, error in (no error)=w959) -> (queue out=w963:refnum<queue>, error out=w958:errorcluster)  [unwired: 1 in, 1 out]
            n503 = Enqueue Element(queue=w962, element=w960, error in (no error)=w958) -> (queue out=w961:refnum<queue>, error out=w957:errorcluster)  [unwired: 1 in, 1 out]
          }
        }
        n504 = Equal?(x=w945, y=T9."Scanning Mode") -> (x = y?=w951:bool)
        n505 = Select(t=Digitizer_StatesMain."Read" ("f"), s=w951, f=Digitizer_StatesMain."SetParam") -> (s? t:f=w948:T4)
      }
      frame "CloseApp" {
        w969 = TRUE
        n506 = call "PXITrigReserve-Unreserve.vi"("error in"=w972, "Mode"=enum16{"Reserve", "Unreserve"}."Unreserve", "FPGA VI Reference In"=w971) -> ("error out"=w973:errorcluster, "FPGA VI Reference Out"=w974:T17)  [unwired: 7 in]
        n507 = xnode "Close FPGA VI Reference"("FPGA VI Reference In"=w974, "error in"=w973) -> ("error out"=w970:errorcluster)
      }
    }
    n508 = call <vilib>:"Share Stop Signal.vi"("set stop (F)"=w821, "channel"=w819) -> ("stop"=w820:bool)
    "nDigiLoopRunning" <- w820
    n509 = call <instrlib>:"Synchronous Latch.vi"("clear"=w838, "set"=w841) -> ("out"=→"Digitizer On":bool)  [unwired: 9 in]
    n510 = Or(x="Stop Digi App", y=w832) -> (x .or. y?=w836:bool)
    n511 = Select(t=u16 0, s="CountReset", f=w827) -> (s? t:f=w826:u16)
    n512 = Select(t=Digitizer_StatesMain."CloseApp", s=w836, f=w833) -> (s? t:f=w834:T4)
    "Digi State" <- w846
  }
  "error out Digi" <- w15
  n513 = timed-loop "Digitizer UI Handle" {
    timing: w42 -> [_]
    timing-out: [_] -> w41
    tunnel: w1 -> [w977]
    stop <- w976 stop-if-true
    n514 = First Call?() -> (First Call?: T/F=w978:bool)
    n515 = node-c288() -> ()  [unwired: 1 in, 1 out]
    n516 = call <extravilib>:"Read.vi"("channel"=w977) -> ("element"=w976:bool)  [unwired: 1 in, 1 out]
    n517 = case shown="True" w978 {
      frame False {
      }
      frame True {
        n518 = property on="Delay(us)" class="DigNum (strict)"("Val(Sgnl)"=sgl 0.0 ("Value (Signaling)")) -> ()  [unwired: 2 in, 2 out]
      }
    }
    n519 = event shown="[1] \"Amplitude Range\": Value Change" {
      selector: _ -> [_ _ _ _]
      dyn-events: _ -> [_ _ _ _]
      timeout: 0 -> [_ _ _ _]
      event Timeout {
        n520 = event-data() -> ()  [unwired: 1 in, 3 out]
      }
      event "Amplitude Range": Value Change {
        n521 = event-data() -> ("NewVal"=w986:cluster{"Slider 1":dbl, "Slider 1":dbl})  [unwired: 1 in, 5 out]
        n522 = Unbundle(w986) -> ("Slider 1"=w985:dbl, "Slider 1"=w984:dbl)
        n523 = Less?(x=w985, y=w984) -> (x < y?=w983:bool)
        n524 = case shown="True" w983 {
          tunnel: w985 -> [_ w988]
          tunnel: w984 -> [_ w987]
          frame False {
          }
          frame True {
            n525 = property on="Waveform [LIVE]" class="WFGraph (strict)"("YScale.Minimum"=w988, "YScale.Maximum"=w987) -> ()  [unwired: 2 in, 2 out]
          }
        }
      }
      event "FineDelayControl": Value Change {
        n526 = event-data() -> ("OldVal"=w992:dbl, "NewVal"=w993:dbl)  [unwired: 1 in, 4 out]
        n527 = Subtract(x=w993, y=w992) -> (x-y=w991:dbl)
        n528 = property on="Delay(us)" class="DigNum (strict)"() -> ("Value"=w990:sgl)  [unwired: 2 in, 2 out]
        n529 = Add(x=w991, y=w990) -> (x+y=w989:dbl)
        n530 = property on="Delay(us)" class="DigNum (strict)"("Value"=w989) -> ()  [unwired: 2 in, 2 out]
      }
      event "Delay_Scroll_Range", "Delay(us)": Value Change {
        w996 = 0.1 ("Scale.Range:Increment")
        n531 = event-data() -> ()  [unwired: 1 in, 6 out]
        n532 = property on="Delay(us)" class="DigNum (strict)"() -> ("Value"=w994:sgl)  [unwired: 2 in, 2 out]
        n533 = Subtract(x=w994, y="Delay_Scroll_Range") -> (x-y=w998:dbl)
        n534 = Add(x=w994, y="Delay_Scroll_Range") -> (x+y=w997:dbl)
        n535 = property on="FineDelayControl" class="Slide (strict)"("Scale.Increment"=w996, "Scale.MinorInc"=w996, "Scale.Minimum"=w998, "Scale.Maximum"=w997, "Value"=w994) -> ()  [unwired: 2 in, 2 out]
      }
    }
    n536 = node-c288() -> ()  [unwired: 1 in, 1 out]
  }
  n537 = node-c288(w41) -> ()  [unwired: 1 out]
  n538 = while {
    shift-right: [w1001] -> _
    shift-left: Data_Save_State."Idle" -> [w1015]
    shift-right: [w1007] -> _
    shift-left: w8 -> [w1008]
    shift-right: [w1006] -> _
    shift-left: w22 -> [w1004]
    shift-right: [w1005] -> _
    shift-left: w21 -> [w1003]
    shift-right: [w999] -> _
    shift-left: w7 -> [w1000]
    stop <- w1002 stop-if-true
    n539 = case shown="\"Close File\"" w1015 {
      tunnel: [w1018 Data_Save_State."Write Attributes" Data_Save_State."Append Data" w1093 Data_Save_State."Idle" Data_Save_State."Idle"] -> w1014
      tunnel: [w1022 _ _ _ TRUE ("Ext/nViTrig") w1107] -> w1010
      tunnel: [_ _ _ _ _ w1107] -> w1002
      tunnel: [_ _ TRUE ("Elements Added?") TRUE ("Elements Added?") _ _] -> w1009
      tunnel: w1008 -> [w1026 w1034 w1067 w1076 w1101 w1111]
      tunnel: [w1026 w1033 w1066 w1088 w1100 w1110] -> w1007
      tunnel: [w1024 w1032 w1065 w1085 w1097 w1106] -> w1006
      tunnel: [w1025 w1031 w1064 w1086 w1096 w1105] -> w1005
      tunnel: w1004 -> [w1024 _ w1068 w1085 w1099 w1109]
      tunnel: w1003 -> [w1025 _ w1064 w1087 w1098 w1108]
      tunnel: w1000 -> [w1023 w1028 w1037 w1080 w1094 w1103]
      tunnel: [w1023 w1028 w1037 w1079 w1094 w1103] -> w999
      frame "Idle", Default {
        n540 = Select(t=Data_Save_State."Open File", s="Open File", f=Data_Save_State."Idle") -> (s? t:f=w1027:T5)
        n541 = Select(t=Data_Save_State."Close File", s="Done Recording", f=w1027) -> (s? t:f=w1018:T5)
        n542 = First Call?() -> (First Call?: T/F=w1022:bool)
      }
      frame "Open File" {
        n543 = call "H5_RefOpen.vi"("error in (no error)"=w1034, "Filename"="FileName", "File Directory"="File Store Directory") -> ("error out"=w1033:errorcluster, "HDF5 Dataset Ref out"=w1031:T11, "HDF5 Ref out"=w1032:T11)  [unwired: 6 in]
      }
      frame "Write Attributes" {
        n544 = local read "Time Division"() -> (w1054:u8)
        n545 = local read "Sampling Frequency (Hz)"() -> (w1052:u64)
        n546 = local read "Speed Control (mm/s)"() -> (w1058:sgl)
        n547 = local read "Scan Time (Approx.)"() -> (w1045:string)
        n548 = Power Of 2(x=w1054) -> (2^x=w1055:dbl)
        n549 = local read "Waves per Pixel"() -> (w1048:u32)
        n550 = local read "Y Step Size (R)"() -> (w1043:sgl)
        n551 = local read "X Step Size (R)"() -> (w1044:sgl)
        n552 = local read "Amplitudes"() -> (w1050:dbl[])
        n553 = local read "Offset Factor"() -> (w1049:dbl)
        n554 = local read "Pixel Count"() -> (w1057:i32)
        n555 = local read "Record Size"() -> (w1046:u16)
        n556 = local read "Scan Mode"() -> (w1059:enum16{"Raster", "Serpentine"})
        n557 = local read "Line Count"() -> (w1056:i32)
        n558 = local read "Delay(us)"() -> (w1042:sgl)
        n559 = Divide(x=1600000000.0 ("Sample Rate"), y=w1055) -> (x/y=w1047:dbl)
        n560 = local read "X Start"() -> (w1063:sgl)
        n561 = local read "Y Start"() -> (w1061:sgl)
        n562 = local read "X End"() -> (w1062:sgl)
        n563 = local read "Y End"() -> (w1060:sgl)
        n564 = local read "Gain"() -> (w1051:dbl)
        n565 = call "H5_WriteAttr.vi"("HDF5 Ref In"=w1068, "X Start"=w1063, "X End"=w1062, "Y Start"=w1061, "Y End"=w1060, "Scan Mode"=w1059, "Speed Control (mm/s)"=w1058, "error in (no error)"=w1067, "Scan Time (Approx.)"=w1045, "Pixel Count"=w1057, "X Step Size (R)"=w1044, "Line Count"=w1056, "Y Step Size (R)"=w1043, "Gen Sampling Rate"=w1052, "Amplitudes (V)"=w1050, "Offset"=w1049, "Gain"=w1051, "Waves per Pixel"=w1048, "Record Size"=w1046, "Delay(us)"=w1042, "Sampling Freq (Hz)"=w1047, "Temperature"="Temperature (C)", "Remarks"="Remarks", "Transducer Freq(Hz)"="Transducer Freq (Hz)", "Immersion Medium"="Immersion Medium") -> ("HDF5 Ref Out"=w1065:T11, "error out"=w1066:errorcluster)  [unwired: 1 in]
      }
      frame "Append Data" {
        n566 = Dequeue Element(queue=w1080, timeout in ms (-1)=150, error in (no error)=w1076) -> (queue out=w1079:refnum<queue>, element=w1077:T10, timed out?=w1078:bool, error out=w1075:errorcluster)
        n567 = Unbundle By Name(w1077) -> ("Wave"=w1074:i16[], "Wave Count"=w1073:u32)
        n568 = Increment(x=w1073) -> (x+1=w1070:u32)
        n569 = Compound Arithmetic op=AND("Record Data", invert w1078) -> (w1089:bool)
        n570 = call "AppendWaveToFile.vi"("Waveform"=w1074, "error in (no error)"=w1075, "Append?"=w1089, "HDF5 Dataset Ref"=w1087) -> ("error out"=w1088:errorcluster, "HDF5 Dataset out"=w1086:T11)  [unwired: 5 in, 1 out]
        n571 = local read "Total Pixels"() -> (w1084:i32)
        n572 = local read "Done Recording"() -> (w1071:bool)
        n573 = Greater Or Equal?(x=w1070, y=w1084) -> (x >= y?=w1082:bool)
        "No Trig Miss" <- w1082
        n574 = Or(x=w1071, y=w1082) -> (x .or. y?=w1083:bool)
        n575 = Select(t=Data_Save_State."Close File", s=w1083, f=Data_Save_State."Append Data") -> (s? t:f=w1093:T5)
      }
      frame "Close File" {
        w1096 = T11 refnum items=["HDF5 Ref"] ("HDF5 Dataset out")
        w1097 = T11 refnum items=["HDF5 Ref"] ("HDF5 Ref out")
        n576 = call "H5_CloseFile.vi"("error in (no error)"=w1101, "HDF5 Dataset Ref"=w1098, "HDF5 Ref"=w1099) -> ("error out"=w1100:errorcluster)  [unwired: 8 in]
      }
      frame "Close App" {
        w1105 = T11 refnum items=["HDF5 Ref"] ("HDF5 Dataset out")
        w1106 = T11 refnum items=["HDF5 Ref"] ("HDF5 Ref out")
        w1107 = TRUE ("Ext/nViTrig")
        n577 = call "H5_CloseFile.vi"("error in (no error)"=w1111, "HDF5 Dataset Ref"=w1108, "HDF5 Ref"=w1109) -> ("error out"=w1110:errorcluster)  [unwired: 8 in]
      }
    }
    n578 = call <instrlib>:"Synchronous Latch.vi"("clear"=w1010, "set"=w1009) -> ("out"=→"File Open?":bool)  [unwired: 9 in]
    n579 = Select(t=Data_Save_State."Close App" ("f"), s="Stop File App", f=w1014) -> (s? t:f=w1001:T5)
    "FileStore State" <- w1015
  }
